vi "BatteryCal FTS.vi"() -> ()   [LabVIEW 2013]
uses:
  Controls/Gen2 FT states.ctl
  SubVI/ESTOP CONTROL.ctl
  Controls/InfoPacket.ctl
  Controls/Target RF Channel.ctl
  <vilib>/Utility/error.llb/DialogType.ctl
  Controls/LocalVars.ctl
  Controls/Iniial Device Programming.ctl
  SubVI/ProgramStageControl.ctl
  Controls/Batt Cap Steps.ctl
  Controls/Support Script.ctl
  Controls/Serial Table.ctl
  Controls/Device Information.ctl
  Controls/Loading.ctl
  Controls/Load Step.ctl
  Controls/Mark10 Config.ctl
  Controls/PID parameters.ctl
  Controls/Channels.ctl
  RxTx/XceiverStates.ctl
  RxTx/XceiverCmds.ctl
  Controls/Mark10 states.ctl
  Controls/Gen2 FT Globals.vi
  <vilib>/Utility/file.llb/Write To Spreadsheet File (I64).vi
  <vilib>/Utility/config.llb/Write Key (String).vi
  <vilib>/Utility/config.llb/NI_LVConfig.lvlib
panel:
  out "Transceiver Channel:":u8
  out "DUT Serial Number":u32
  in  "A2 Delay (ms)":i16=500 min=-1 step=1
  in  "Save EEPROM Data":bool caption="DevOFF"
  out "EEPROM Data":i32[][](array[numeric])
  in  "Close Xsceiver":bool
  in  "Scan Channels":bool caption="DevOFF"
  in  "Clear Message":bool
  out "Rev String":string
  in  "Target Channel:":T1="5"
  in  "mSec":u8=1 min=1 max=50 step=1
  in  "Set Wndow":bool caption="DevOFF"
  in  "Get Window":bool caption="DevOFF"
  out "ADBatt":u16
  out "BattVolts":dbl format="%_3g"
  out "BatteryCapState":i8
  out "Batt280":i32
  out "Batt310":i32
  out "Accelerometer sample size":i32
  out "Base Accels":dbl[][](array[numeric])
  out "Six Plane Accels":dbl[][](array[numeric])
  in  "Reset Device":bool=TRUE
  in  "CaptureButton":bool
  out "Message":string
  out "AssemScore":i32
  out "PCB Score":i32
  out "GAINC Reprogram?":bool
  out "Three Failed Tests":dbl
  in  "Mark-10 COM Port":refnum<visa-resource-name>="COM1"
  in  "Eng-Result# :":u32 max=268435455
  in  "Start Channel:":string(combo)="3"
  in  "Brand:":string(combo)
  in  "DeviceType:":string(combo)="SYK-TRCR01"
  out "Device Parameters":T2 {"ASICtrim" format="%02x"}
  out "Device ON?":bool
  in  "Start":bool
  out "SoftwareVersion":string="SW-03004-002"
  out "Adj.Data":dbl[](array[numeric])
  out "RawData":u16[](array[numeric]) caption="RawData\n      S3         S4           S5         S6         S7          S8          S9          B"
  in  "Operator":string caption="Operator Name:"
  out "DeviceID:":u32
  out "Current Time:":timestamp=timestamp(3438190648.7035365 s since 1904-01-01) format="%<%I:%M:%S %p\n%m/%d/%Y>T"
  in  "Lot#:":u32
  in  "ClearBuffer":bool
  in  "Exit":bool
  in  "Estop":T3
  in  "Shutdown Dev":bool caption="DevOFF"
  out "Test Result":bool
  in  "States":T4=enum."Initialization"
  out "error out":errorcluster
  # "lbs"
  # "inch"
  # "Mark-10"
  # "Engineering Panel"
  # "OrthoSensor Battery Calibration"
  # "System Messages"
  # "Target Loads\n(lbs)"
  # "Gauge Loads\n(lbs)"
  # "Total Device \nLoads (lbs)"
  # "Device Loads"
  # "Errors"
  # "A (lbs)                  B (lbs)"
  # "A (lbs)                 B (lbs)"
  # "Device"
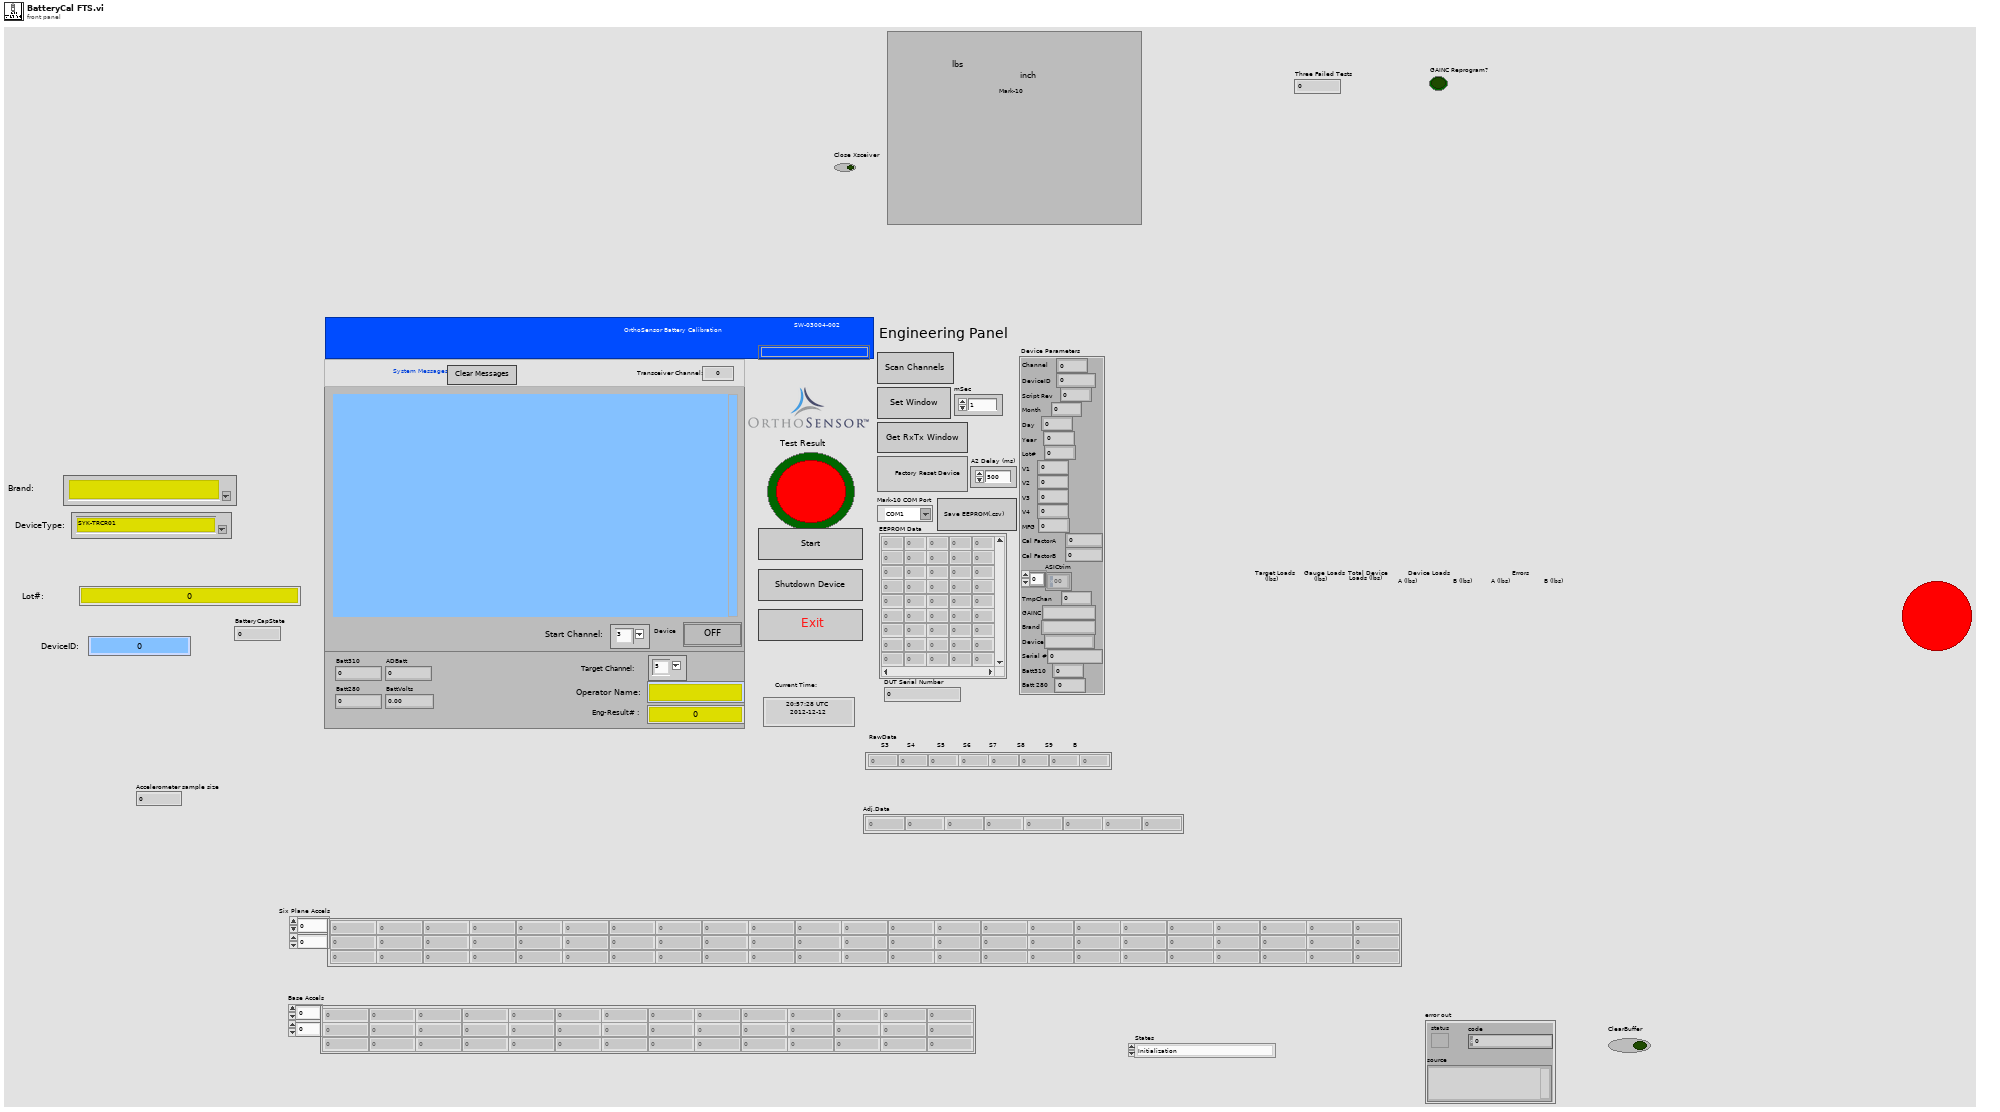
[diagram p1: front panel]
types:
  T1 = typedef "Target RF Channel.ctl" = string
  T2 = typedef "InfoPacket.ctl" = cluster{"Channel":u8, "DeviceID":u32, "Script Rev":u8, "Month":u8, "Day":u8, "Year":u8, "Lot#":u32, "V1":u16, "V2":u16, "V3":u16, "V4":u16, "MFG":u8, "Cal FactorA":u8, "Cal FactorB":u8, "ASICtrim":u8[], "TmpChan":u8, "GAINC":string, "Brand":string, "Device":string, "Serial #":u64, "Batt310":u16, "Batt 280":u16}
  T3 = typedef "ESTOP CONTROL.ctl" = bool
  T4 = typedef "Gen2 FT states.ctl" = enum16{"---------SETUP-------", "Initialization", "Read Support Data", "Initialize Mark-10", "Initialize Transceiver", "------UTILITIES------", "Change DUT Channel", "Find RxTx Window", "Reset Device", "Scan Channels", "Read Serial Lookup", "Shutdown Device", "ESTOP", "--------USER---------", "Timeout", "-----PROGRAM-----", "Program Device", "------MARK10--------", "Go Home", "MoveUp", "MoveDown", "Goto Load", "Goto Position", "Stop Motor", "---------TESTS--------", "Start Test", "Angle Test", "Load Test", "Load Accuracy Test", "Battery Test", "------RESULTS-------", "End Test", "Display Result", "--------EXIT--------", "Exit"}
  T5 = typedef "XceiverStates.ctl" = enum16{"Initialize", "Rx", "Tx", "Raw Mode", "Clear Buffer", "ClearEcho", "Read Buffer", "Close"}
  T6 = typedef "LocalVars.ctl" = cluster{"Message":string, "Homed?":bool, "NextState":T4, "G.Load":dbl, "G.Position":dbl, "Load#":i32, "[G.Loads]":dbl[], "[TotalLoads]":dbl[], "[Errors]":dbl[][], "ZeroWait":u32, "Results":dbl[], "DwellWait":bool, "Test Result":bool, "[CondyleLoads]":dbl[][], "[Max]":dbl[], "[Min]":dbl[], "Valid String?":bool, "ScanTime":timestamp, "ScannedString":string, "LabelDevID":u32, "MfgDate":timestamp, "[EEPROM Cmds]":u8[][], "[CalData]":u8[][], "[A/Ds]":dbl[][], "[A/Dmax]":dbl[], "[A/Dmin]":dbl[], "BattMax":dbl, "BattMin":dbl, "DwellTime":i32, "PendingDeviceType":string, "Zero G.load":dbl, "GAINC Value":string, "Programming Step":T7, "Front Panel Program?":bool, "Final Program?":bool, "PCB Score":i32, "AssyScore":i32, "Pass/Fail #":string, "Result String":string, "Programming Mode":T8, "Angle Test Step":enum16{"Initialize", "Get X", "Get Y", "Get Z", "Next Test"}, "Accel Values":dbl[][], "Shutdown Counter":u32, "V1":i32, "V2":i32, "V3":i32, "V4":i32, "EEPROM Data":i32[][], "Counter":i32, "Page#":i32, "Timer":timestamp, "Use Mark10?":bool, "Eng-Result#":u32, "DUT Serial #":i32, "Scroll Message?":bool, "Clear Message":bool, "Batt Test Step ":T9, "RXTX Window Found?":bool, "Shutdown First Call?":bool, "A2 Delay (msec)":i16, "Support Script":T10, "Serial Table":T11, "Target Information":T12, "Operator":string, "COM Port":string, "Config Path":path, "Tx Array":u8[], "DUT Parameters":T2, "FTS Main?":bool, "Loading":T13, "Software Version":string, "Correction Factor":string, "Second Load Test":bool, "Acc Loads":dbl[][], "Mark10 Config":T15, "Channels":T17, "Channel EEPROM":i32[][], "Load Notes":string[], "Engr Log?":bool, "Time":timestamp[], "Program Retry":bool, "Operator Channel":string, "Target Channel ":string, "New Data Program":bool}
  T7 = typedef "Iniial Device Programming.ctl" = enum16{"Load EEPROM", "Send First A1", "Send EEPROM", "Send A1", "Check EEPROM Echo", "Verify transmission", "Programming Successful", "Programming Failed"}
  T8 = typedef "ProgramStageControl.ctl" = enum16{"Initial Program", "GainC", "Scales"}
  T9 = typedef "Batt Cap Steps.ctl" = enum16{"Initialize", "Collect 2.8 Volts", "Collect 3.1 Volts", "Check Results"}
  T10 = typedef "Support Script.ctl" = cluster{"Script #":string, "Script Revision":string, "[OEMs]":string[], "[[DeviceTypes]]":string[][], "[[DeviceTypesVals]]":u16[][], "[[List of Errors]]":string[][], "Default GAINC":string, "[[ASICtrims]]":u8[][], "ID For Echo":string, "Condyle A CalFactor":i32, "Condyle B CalFactor":i32, "[OEMs Prefix]":string[], "Packet ID 18":string, "[[Force Table Load Test]]":dbl[][], "[[Force Table AccurTest]]":dbl[][]}
  T11 = typedef "Serial Table.ctl" = cluster{"Serial File Path":path, "[[Serial Lookup Table]]":string[][], "Serial Device Info":string[], "Valid Serial?":bool}
  T12 = typedef "Device Information.ctl" = cluster{"Target Brand":string, "Target DeviceType":string, "Target Serial#":i32, "Target Lot#":u32, "Target DevID":u32, "Target Channel":u8}
  T13 = typedef "Loading.ctl" = cluster{"[Forces]":dbl[], "[Dwell]":dbl[], "Loading Step":T14}
  T14 = typedef "Load Step.ctl" = enum16{"Initialize Test", "Go Home", "Detect Dev Surface", "Wait to zero Device", "Zero Device", "Do Test", "Test Result"}
  T15 = typedef "Mark10 Config.ctl" = cluster{"H2S%":dbl[], "H2S Speed":dbl[], "H to S":dbl, "Home Speed":dbl, "LoadWin":dbl, "Load Speed":dbl, "PID":T16}
  T16 = typedef "PID parameters.ctl" = cluster{"Kp":dbl, "Kd":dbl, "Ki":dbl}
  T17 = typedef "Channels.ctl" = cluster{"Transceiver Ch":u8, "Operating Ch":u8, "Start Ch":u8}
  T18 = typedef "DialogType.ctl" = u16
  T19 = enum8{"Enabled", "Disabled", "Disabled and Grayed Out"}
  T20 = enum16{"None", "On Hover", "On Key Focus", "On Hover or Key Focus"}
  T21 = typedef "Mark10 states.ctl" = enum16{"Initialize", "Go Home", "Move Up", "Move Down", "Stop @ Load", "Read Status", "Goto Position", "Goto Device Surface", "Stop Motor", "Shutdown", "Exit"}
  T22 = typedef "XceiverCmds.ctl" = enum8{"Get Window", "Set Window", "Load&Xmit", "Find Window", "Load CC1101", "Blink LED1", "Blink LED2", "Gen2 Mode", "Request Rev", "Gen2 Mode & Req Rev", "Load Device Settings", "Reset Xceiver", "Set Channel", "Read Channel"}
  T23 = cluster{"Shift":bool, "Ctrl":bool, "Alt":bool, "Cmd":bool, "Opt":bool}
  T24 = typedef "Scanned Data.ctl" = cluster{"DeviceID":u32, "Mfg Date":timestamp, "ScannedIn":bool, "Lot#":u32}
  T25 = typedef "LVRectTypeDef.ctl" = cluster{"Left":i16, "Top":i16, "Right":i16, "Bottom":i16}
  T26 = typedef "DeviceInfo.ctl" = cluster{"DevInfo":T2, "Mfg Date":timestamp, "[CalData]":u8[][], "[DevData]":u8[], "GotCal":bool, "CustomCal?":bool, "Packet#":i32}
  T27 = typedef "NI_LVConfig.lvlib/Config Data RefNum.ctl" = refnum<k1>
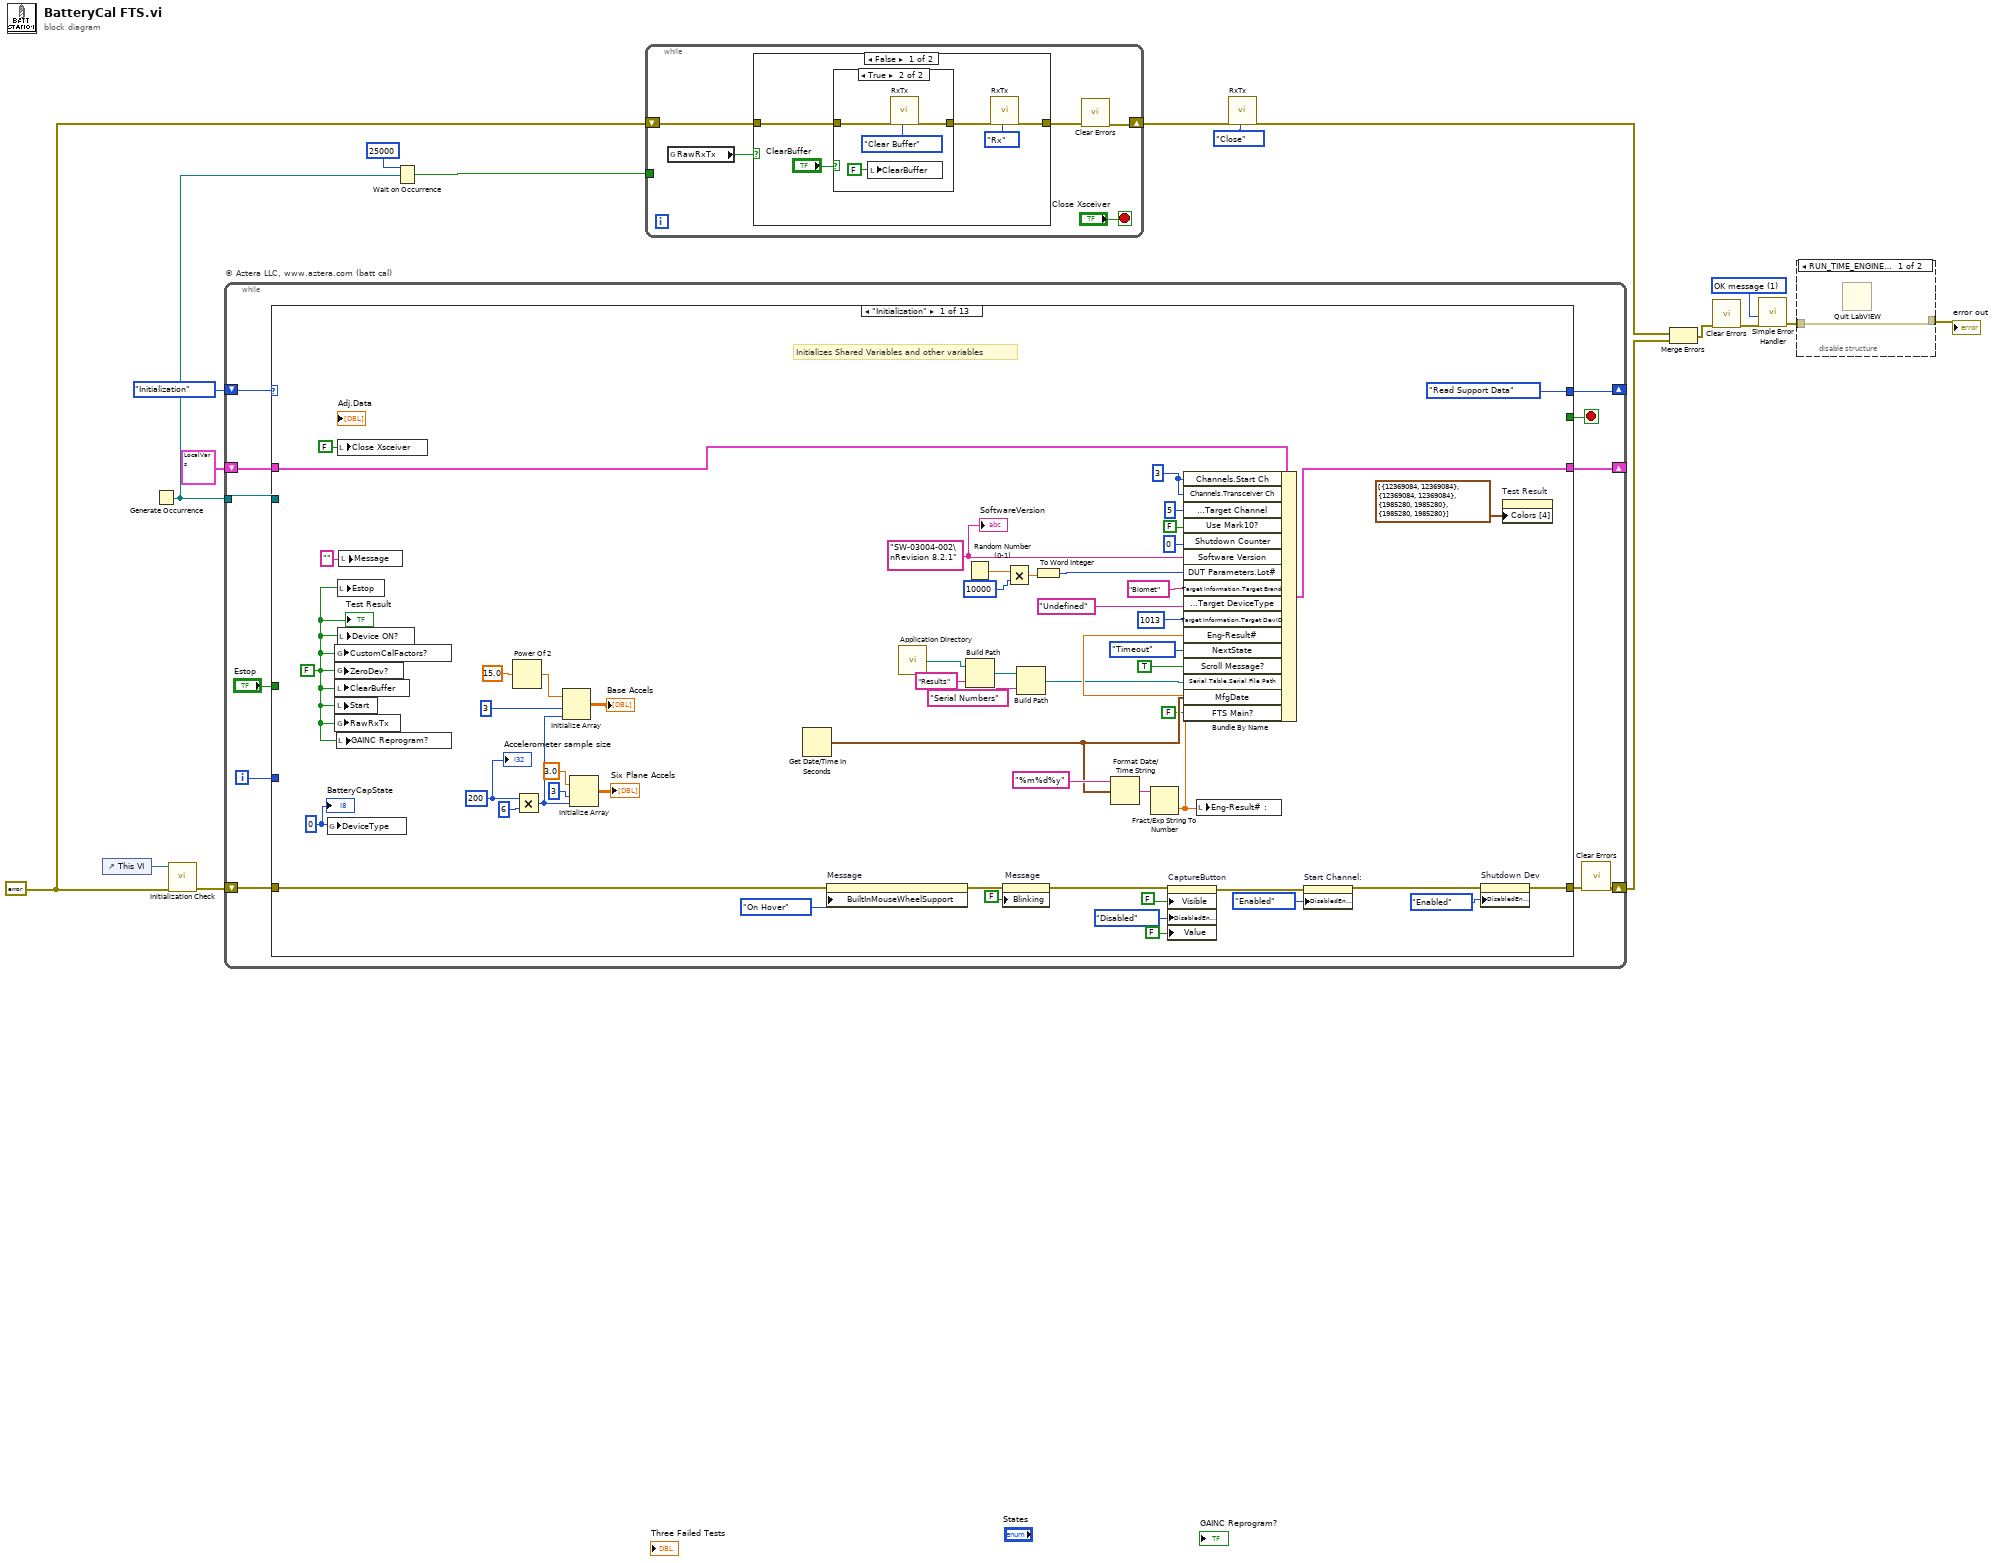
[diagram p0: block diagram]
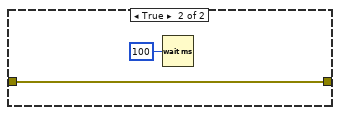
[diagram p3: hidden frame]
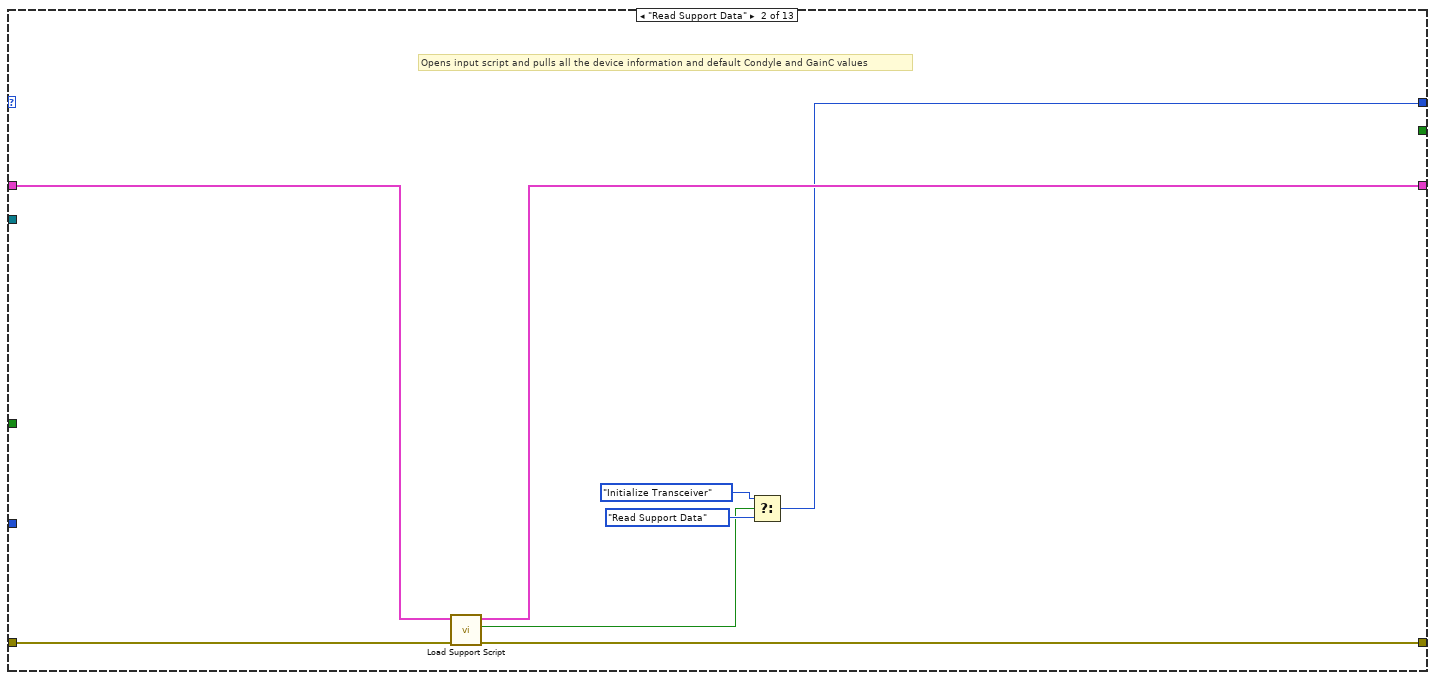
[diagram p5: hidden frame]
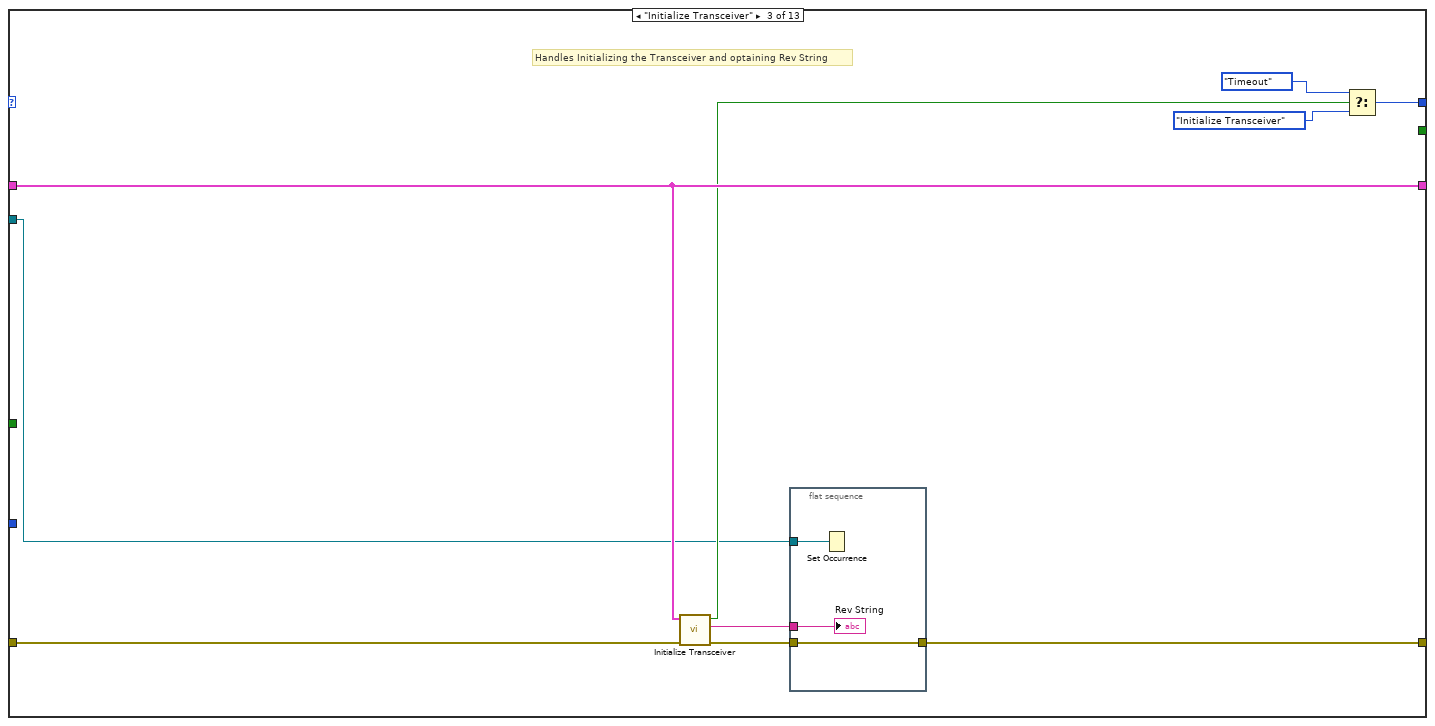
[diagram p6: hidden frame]
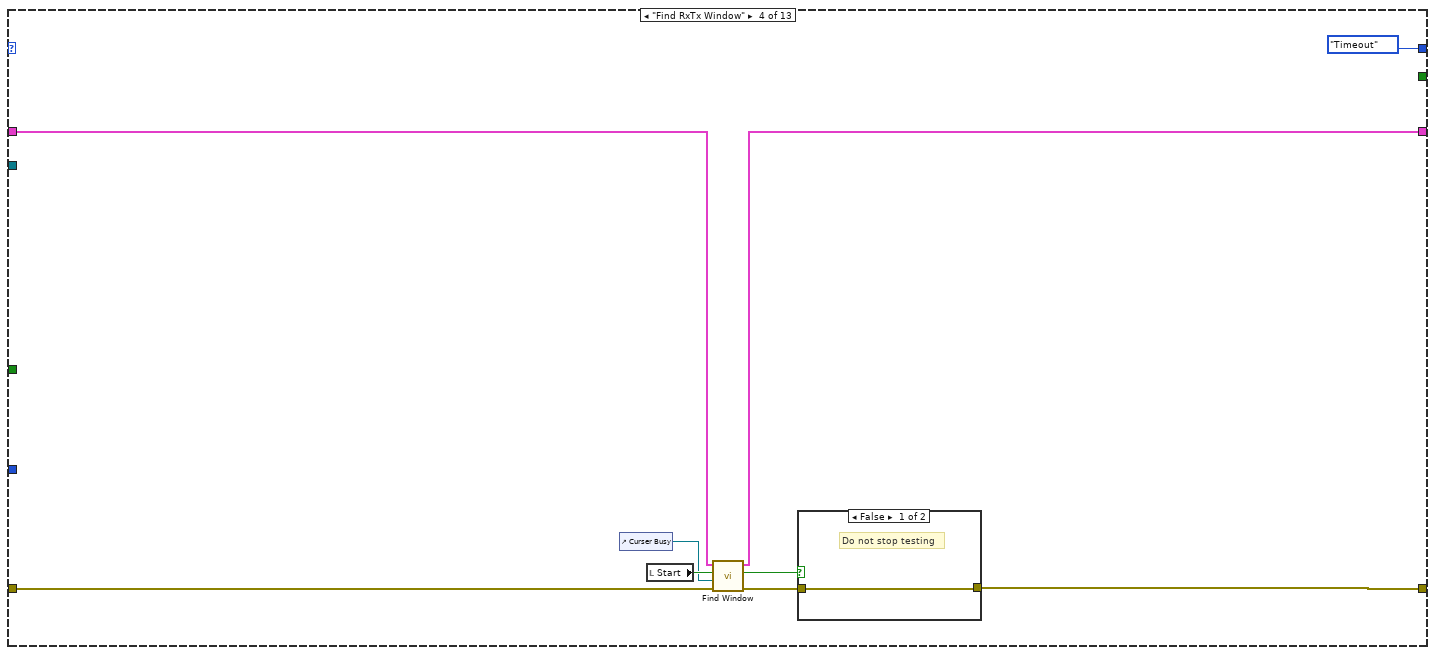
[diagram p7: hidden frame]
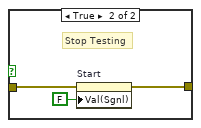
[diagram p8: hidden frame]
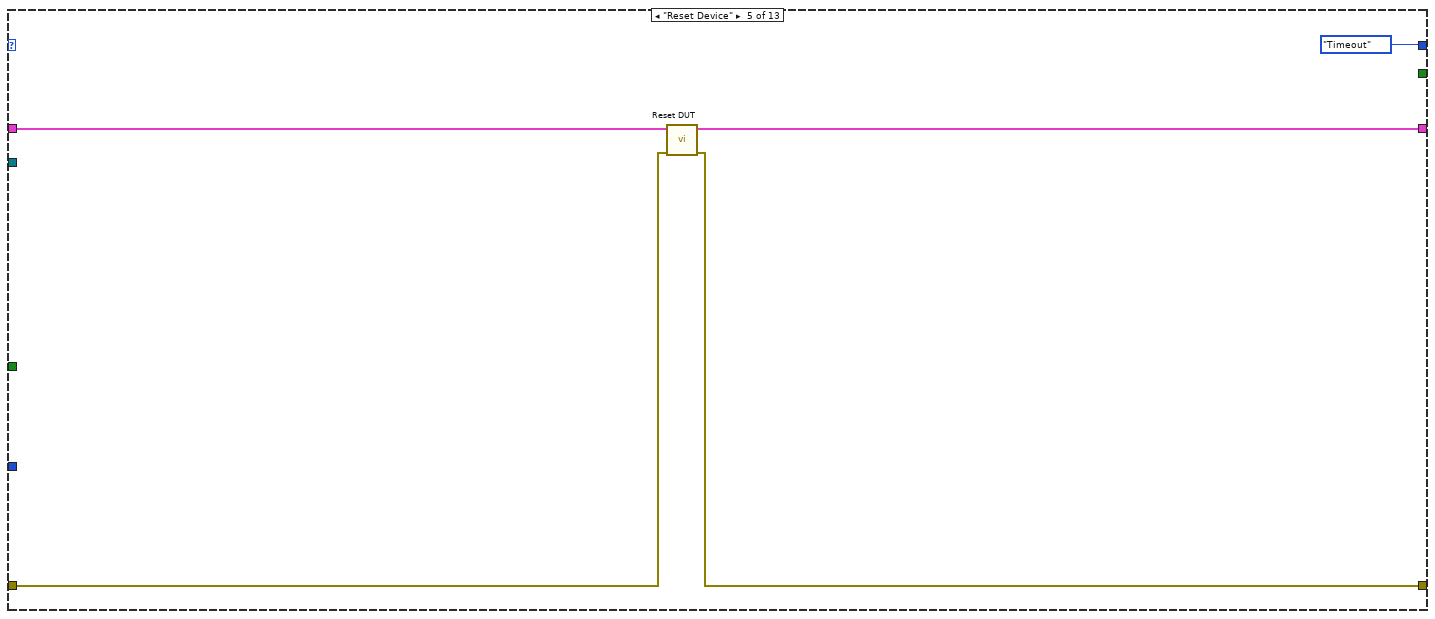
[diagram p9: hidden frame]
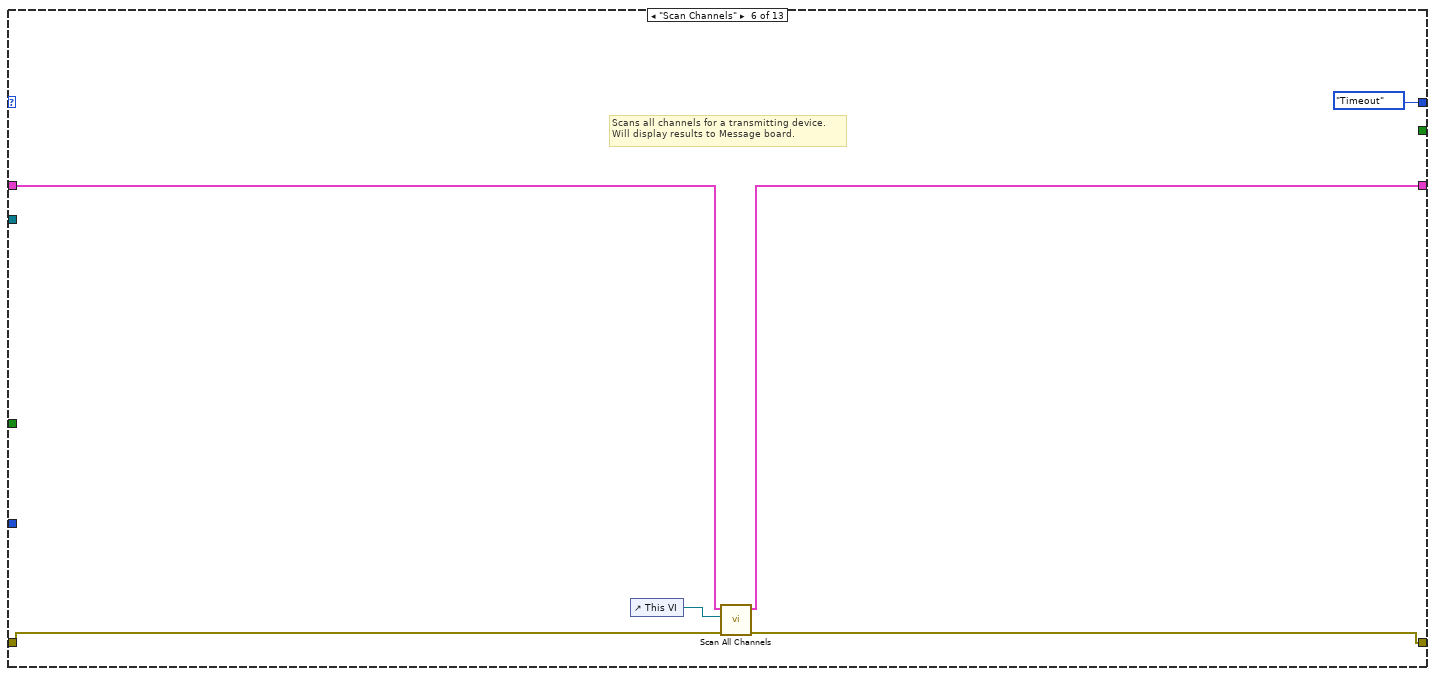
[diagram p10: hidden frame]
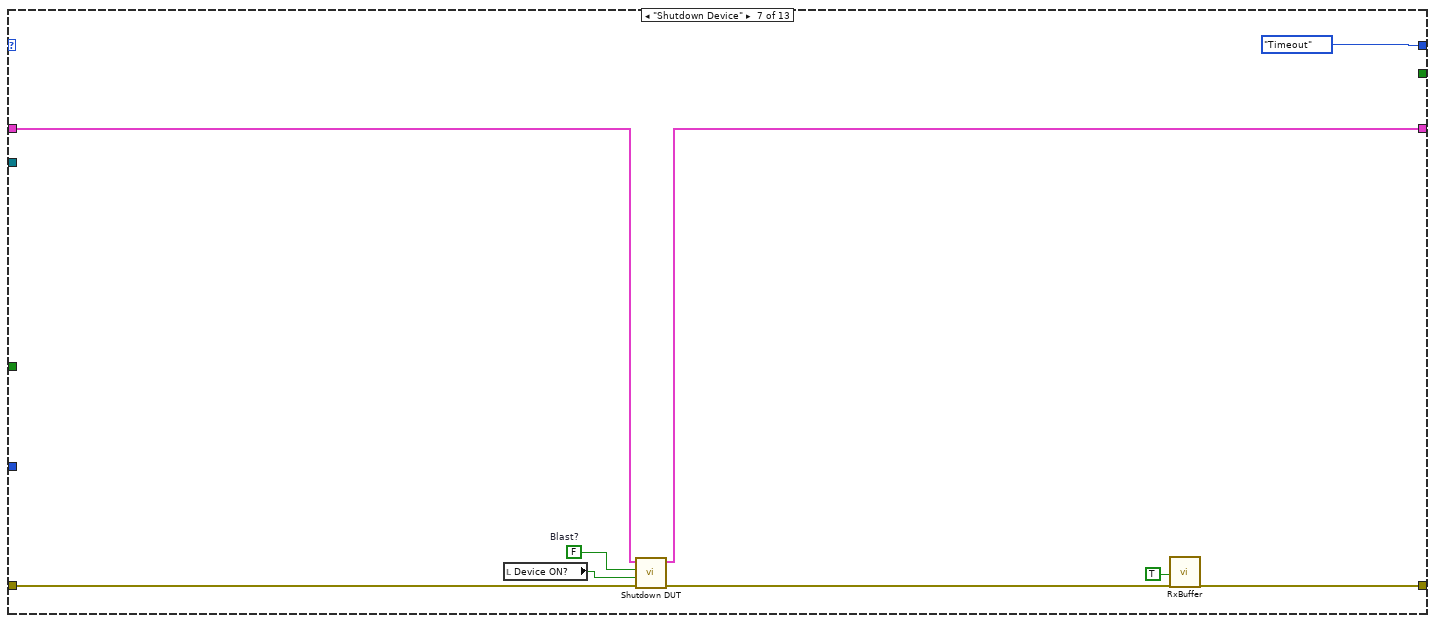
[diagram p11: hidden frame]
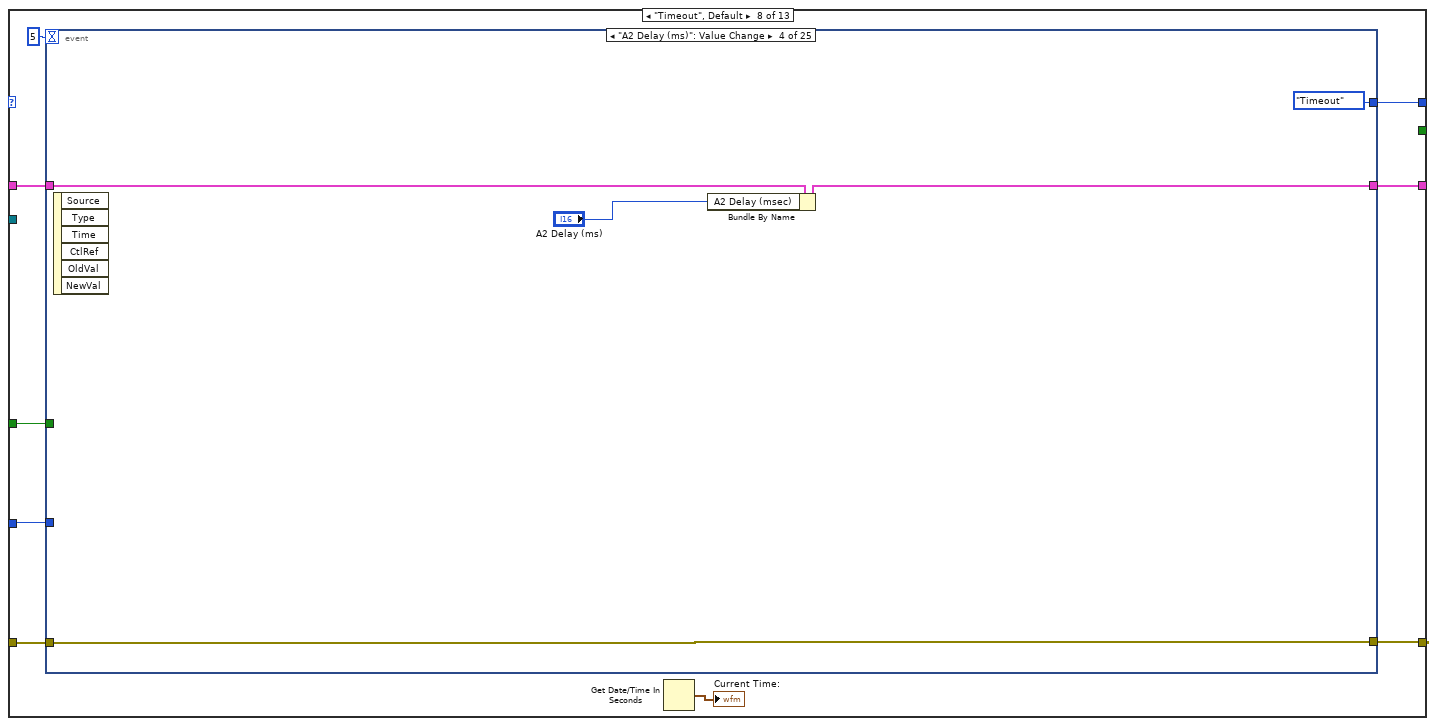
[diagram p12: hidden frame]
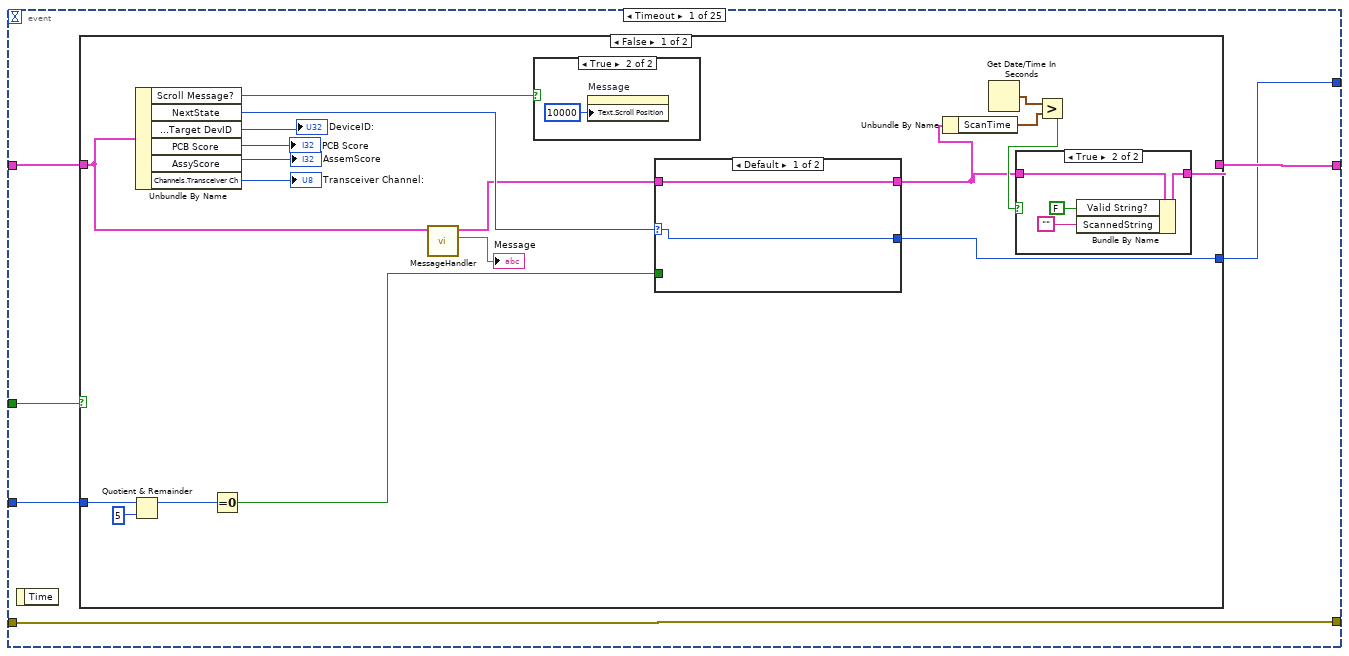
[diagram p13: hidden frame]
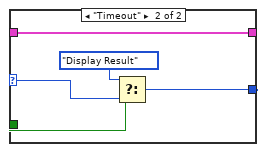
[diagram p16: hidden frame]
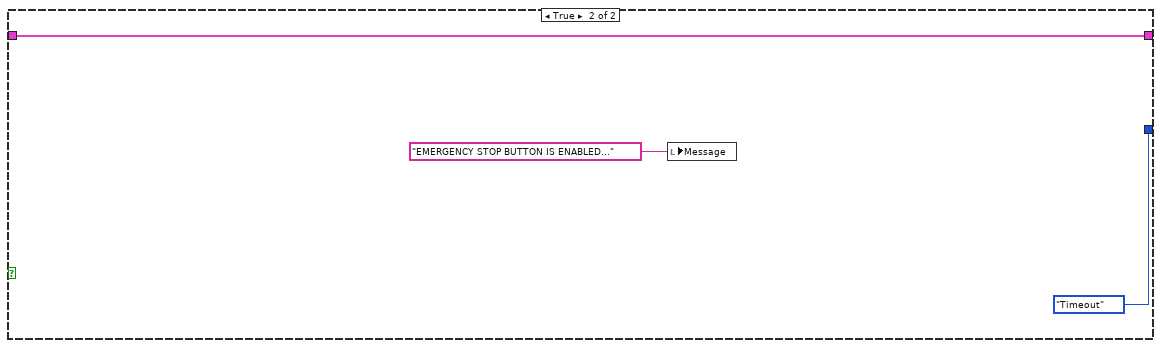
[diagram p17: hidden frame]
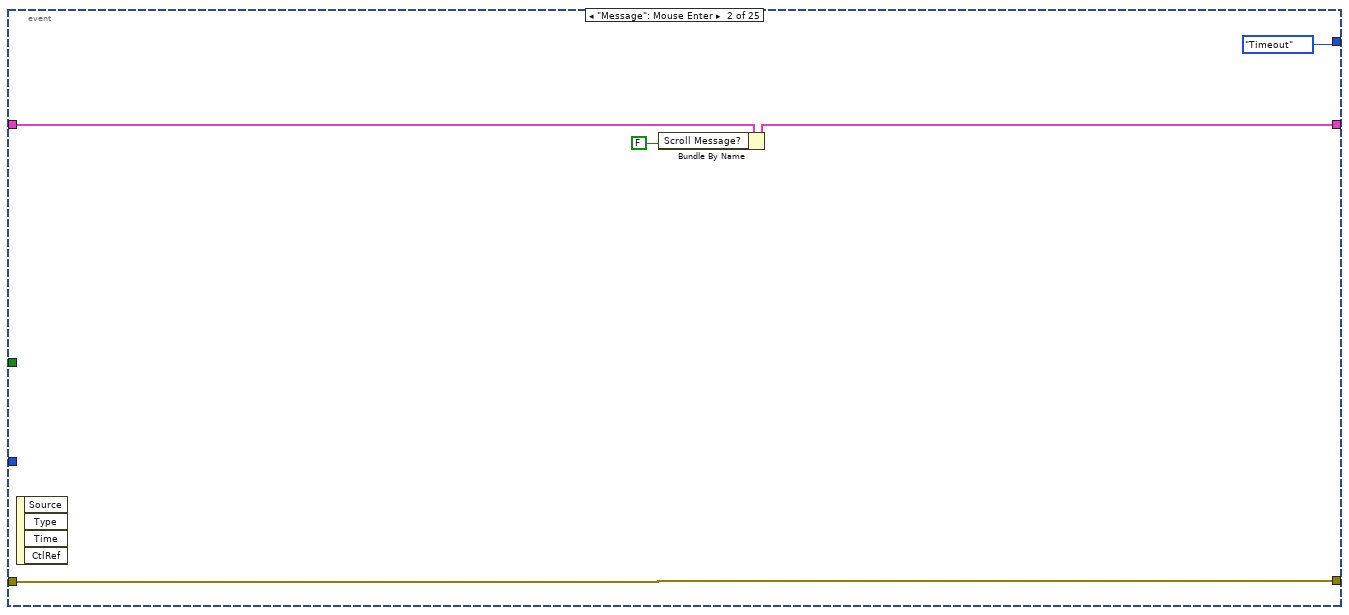
[diagram p18: hidden frame]
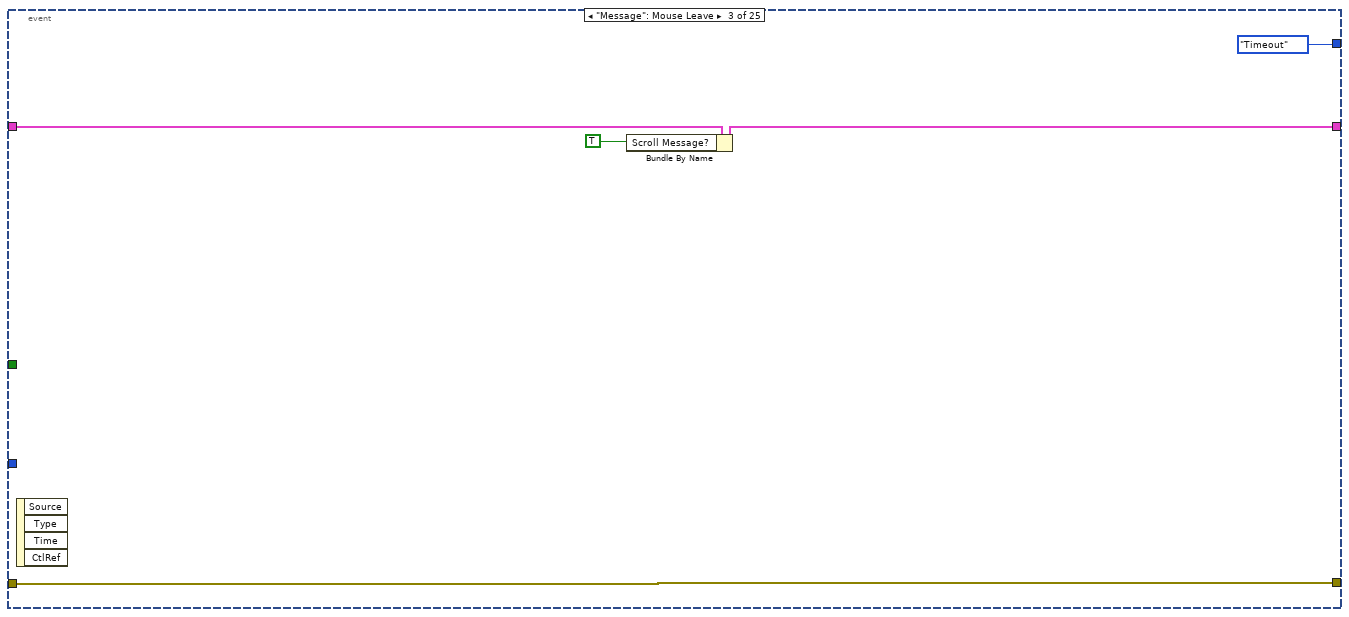
[diagram p19: hidden frame]
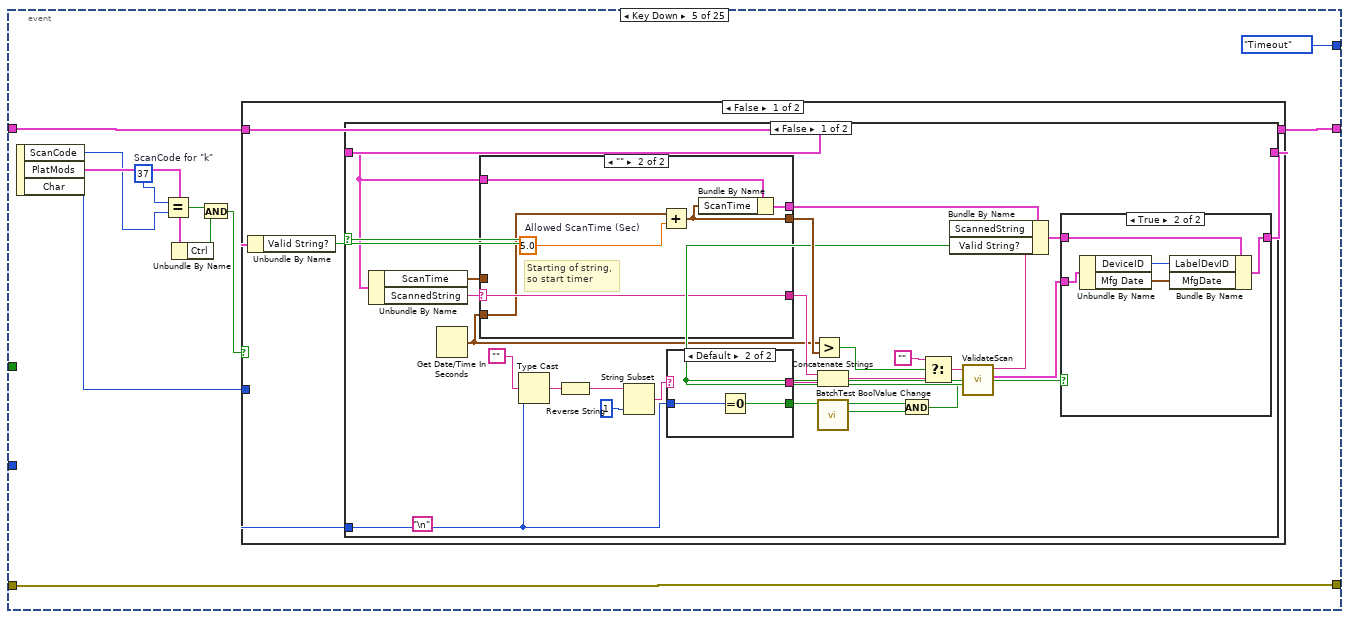
[diagram p20: hidden frame]
diagram:
  w12 = T18 1 items=["no dialog", "OK message", "continue or stop message", "OK message + warnings", "continue/stop + warnings"] ("type of dialog (OK msg:1)")
  w3 = errorcluster {"status"=FALSE, "code"=0, "source"=""} ("error in (no error)")
  n1 = control-ref of="This VI"() -> (w7:refnum<vi>)
  n2 = Generate Occurrence() -> (w15:refnum<k4>)
  n3 = call "Initialization Check.vi"("error in (no error)"=w3, "VI in"=w7) -> ("error out"=w6:errorcluster)  [unwired: 9 in]
  n4 = while "© Aztera LLC, www.aztera.com (batt cal)" {
    shift-right: [w21] -> _
    shift-left: T6 {"Message"="", "Homed?"=FALSE, "NextState"=enum."Scan Channels", "G.Load"=0.0, "G.Position"=0.0, "Load#"=0, "[G.Loads]"=[], "[TotalLoads]"=[], "[Errors]"=[], "ZeroWait"=0, "Results"=[], "DwellWait"=FALSE, "Test Result"=FALSE, "[CondyleLoads]"=[], "[Max]"=[], "[Min]"=[], "Valid String?"=FALSE, "ScanTime"=timestamp(0 s since 1904-01-01), "ScannedString"="", "LabelDevID"=0, "MfgDate"=timestamp(0 s since 1904-01-01), "[EEPROM Cmds]"=[], "[CalData]"=[], "[A/Ds]"=[], "[A/Dmax]"=[], "[A/Dmin]"=[], "BattMax"=0.0, "BattMin"=0.0, "DwellTime"=0, "PendingDeviceType"="", "Zero G.load"=0.0, "GAINC Value"="", "Programming Step"=enum."Load EEPROM", "Front Panel Program?"=FALSE, "Final Program?"=FALSE, "PCB Score"=0, "AssyScore"=0, "Pass/Fail #"="", "Result String"="", "Programming Mode"=enum."Initial Program", "Angle Test Step"=enum."Initialize", "Accel Values"=[], "Shutdown Counter"=0, "V1"=0, "V2"=0, "V3"=0, "V4"=0, "EEPROM Data"=[], "Counter"=0, "Page#"=0, "Timer"=timestamp(0 s since 1904-01-01), "Use Mark10?"=FALSE, "Eng-Result#"=0, "DUT Serial #"=0, "Scroll Message?"=FALSE, "Clear Message"=FALSE, "Batt Test Step "=enum."Initialize", "RXTX Window Found?"=FALSE, "Shutdown First Call?"=FALSE, "A2 Delay (msec)"=0, "Support Script"={"Script #"="", "Script Revision"="", "[OEMs]"=[], "[[DeviceTypes]]"=[], "[[DeviceTypesVals]]"=[], "[[List of Errors]]"=[], "Default GAINC"="", "[[ASICtrims]]"=[], "ID For Echo"="", "Condyle A CalFactor"=0, "Condyle B CalFactor"=0, "[OEMs Prefix]"=[], "Packet ID 18"="", "[[Force Table Load Test]]"=[], "[[Force Table AccurTest]]"=[]}, "Serial Table"={"Serial File Path"=path "", "[[Serial Lookup Table]]"=[], "Serial Device Info"=[], "Valid Serial?"=FALSE}, "Target Information"={"Target Brand"="", "Target DeviceType"="", "Target Serial#"=0, "Target Lot#"=0, "Target DevID"=0, "Target Channel"=0}, "Operator"="", "COM Port"="", "Config Path"=path "", "Tx Array"=[], "DUT Parameters"={"Channel"=0, "DeviceID"=0, "Script Rev"=0, "Month"=0, "Day"=0, "Year"=0, "Lot#"=0, "V1"=0, "V2"=0, "V3"=0, "V4"=0, "MFG"=0, "Cal FactorA"=0, "Cal FactorB"=0, "ASICtrim"=[], "TmpChan"=0, "GAINC"="", "Brand"="", "Device"="", "Serial #"=0, "Batt310"=0, "Batt 280"=0}, "FTS Main?"=FALSE, "Loading"={"[Forces]"=[], "[Dwell]"=[], "Loading Step"=enum."Initialize Test"}, "Software Version"="", "Correction Factor"="", "Second Load Test"=FALSE, "Acc Loads"=[], "Mark10 Config"={"H2S%"=[], "H2S Speed"=[], "H to S"=0.0, "Home Speed"=0.0, "LoadWin"=0.0, "Load Speed"=0.0, "PID"={"Kp"=0.0, "Kd"=0.0, "Ki"=0.0}}, "Channels"={"Transceiver Ch"=0, "Operating Ch"=0, "Start Ch"=0}, "Channel EEPROM"=[], "Load Notes"=[], "Engr Log?"=FALSE, "Time"=[], "Program Retry"=FALSE, "Operator Channel"="", "Target Channel "="", "New Data Program"=FALSE} ("State-machine Local Variables") -> [w26]
    shift-right: [w22] -> w17
    shift-left: w6 -> [w27]
    tunnel: w15 -> [w24]
    shift-right: [w19] -> _
    shift-left: Gen2_FT_states."Initialization" ("Current State Out") -> [w18]
    i -> [w25]
    stop <- w20 stop-if-true
    n5 = case shown="\"Initialization\"" w18 {
      tunnel: [w43 w86 w92 w108 w119 w127 w130 w139 w608 w611 w708 w732 w759] -> w28
      tunnel: w27 -> [w33 w91 w101 w107 w120 w128 w135 w140 w609 w612 w707 w744 w765]
      tunnel: w26 -> [w78 w90 w96 w113 w122 w124 w136 w143 w606 w614 w710 w723 w764]
      tunnel: [Gen2_FT_states."Read Support Data" ("Current State Out") w87 w98 Gen2_FT_states."Timeout" ("Current State Out") Gen2_FT_states."Timeout" ("Current State Out") Gen2_FT_states."Timeout" ("Current State Out") Gen2_FT_states."Timeout" ("Current State Out") w144 Gen2_FT_states."Timeout" ("Current State Out") Gen2_FT_states."Timeout" ("Current State Out") Gen2_FT_states."Timeout" ("Current State Out") Gen2_FT_states."Timeout" ("Current State Out") Gen2_FT_states."Exit" ("Current State Out")] -> w19
      tunnel: w25 -> [_ _ _ _ _ _ _ w142 _ _ _ _ _]
      tunnel: w24 -> [_ _ w94 _ _ _ _ _ _ _ _ _ _]
      tunnel: "Estop" -> [_ _ _ _ _ _ _ w141 _ _ _ _ _]
      tunnel: [w46 w89 w96 w105 w118 w126 w132 w138 w605 w615 w702 w723 w763] -> w21
      tunnel: [_ _ _ _ _ _ _ _ _ _ _ _ TRUE] -> w20
      frame "Initialization" {
        w29 = u8 3 ("Current Channel")
        w55 = "SW-03004-002\nRevision 8.2.1" ("SoftwareVersion")
        w67 = 200
        w76 = u32 0 ("Lot Number")
        w45 = FALSE ("Exit")
        # "Initializes Shared Variables and other variables"
        n6 = global write "Gen2 FT Globals.vi" "DeviceType"(w76) -> ()
        n7 = global write "Gen2 FT Globals.vi" "CustomCalFactors?"(w45) -> ()
        n8 = global write "Gen2 FT Globals.vi" "ZeroDev?"(w45) -> ()
        n9 = local write "ClearBuffer"(w45) -> ()
        n10 = local write "Start"(w45) -> ()
        n11 = global write "Gen2 FT Globals.vi" "RawRxTx"(w45) -> ()
        n12 = local write "GAINC Reprogram?"(w45) -> ()
        n13 = local write "Close Xsceiver"(FALSE ("Close Xsceiver")) -> ()
        n14 = local write "Estop"(w45) -> ()
        n15 = local write "Device ON?"(w45) -> ()
        n16 = local write "Message"("" ("Message")) -> ()
        n17 = Power Of 2(x=15.0) -> (2^x=w75:dbl)
        n18 = Multiply(x=w67, y=6) -> (x*y=w66:i32)
        n19 = Initialize Array(w75, 3, w66) -> (→"Base Accels":dbl[][])
        n20 = Initialize Array(3.0, 3, w66) -> (→"Six Plane Accels":dbl[][])
        n21 = Get Date/Time In Seconds() -> (seconds since 1Jan1904=w32:timestamp)
        n22 = property on="Message" class="Str"(error in=w33, "BuiltInMouseWheelSupport"=T20."On Hover" ("Built-In Mouse Wheel Support")) -> (error out=w77:errorcluster)  [unwired: 1 in, 1 out]
        n23 = call <vilib>:"Application Directory.vi"() -> ("Application Directory"=w38:path)
        n24 = Random Number (0-1)() -> (number: 0 to 1=w54:dbl)
        n25 = Build Path(base path=w38, name or relative path="Results") -> (appended path=w36:path)
        n26 = property on="Message" class="Str"(error in=w77, "Blinking"=FALSE) -> (error out=w56:errorcluster)  [unwired: 1 in, 1 out]
        n27 = Multiply(x=w54, y=10000) -> (x*y=w53:dbl)
        n28 = Build Path(base path=w36, name or relative path="Serial Numbers") -> (appended path=w34:path)
        n29 = To Word Integer(number=w53) -> (16bit integer=w52:i16)
        n30 = Format Date/Time String(time format string (%c)="%m%d%y", seconds (now)=w32) -> (date/time string=w57:string)  [unwired: 1 in]
        n31 = Fract/Exp String To Number(string=w57) -> (number=w50:dbl)  [unwired: 3 in, 1 out]
        n32 = property on="CaptureButton" class="Bool (strict)"(error in=w56, "Visible"=FALSE, "DisabledEnum"=T19."Disabled" ("Disabled"), "Value"=FALSE ("CaptureButton")) -> (error out=w60:errorcluster)  [unwired: 1 in, 1 out]
        n33 = Bundle By Name(cluster=w78, "Channels.Start Ch"=w29, "Channels.Transceiver Ch"=w29, "Target Information.Target Channel"=u8 5 ("Target Channel"), "Use Mark10?"=FALSE ("FTS Main?"), "Shutdown Counter"=u32 0, "Software Version"=w55, "DUT Parameters.Lot#"=w52, "Target Information.Target Brand"="Biomet", "Target Information.Target DeviceType"="Undefined", "Target Information.Target DevID"=1013, "Eng-Result#"=w50, "NextState"=Gen2_FT_states."Timeout", "Scroll Message?"=TRUE, "Serial Table.Serial File Path"=w34, "MfgDate"=w32, "FTS Main?"=FALSE) -> (w46:T6)
        n34 = local write "Eng-Result# :"(w50) -> ()
        n35 = property on="Start Channel:" class="CmbBox"(error in=w60, "DisabledEnum"=T19."Enabled" ("Disabled")) -> (error out=w44:errorcluster)  [unwired: 1 in, 1 out]
        n36 = property on="Shutdown Dev" class="Bool"(error in=w44, "DisabledEnum"=T19."Enabled" ("Disabled")) -> (error out=w43:errorcluster)  [unwired: 1 in, 1 out]
        n37 = property on="Test Result" class="Bool (strict)"("Colors [4]"=cluster{u32, u32}[] [{12369084, 12369084}, {12369084, 12369084}, {1985280, 1985280}, {1985280, 1985280}]) -> ()  [unwired: 2 in, 2 out]
        "BatteryCapState" <- w76
        "Accelerometer sample size" <- w67
        "SoftwareVersion" <- w55
        "Test Result" <- w45
      }
      frame "Read Support Data" {
        # "Opens input script and pulls all the device information and default Condyle and GainC values"
        n38 = call "Load Support Script.vi"("error in (no error)"=w91, "Data In"=w90) -> ("error out"=w86:errorcluster, "Done?"=w84:bool, "Data Out"=w89:T6)  [unwired: 7 in]
        n39 = Select(t=Gen2_FT_states."Initialize Transceiver" ("Current State Out"), s=w84, f=Gen2_FT_states."Read Support Data") -> (s? t:f=w87:T4)
      }
      frame "Initialize Transceiver" {
        # "Handles Initializing the Transceiver and optaining Rev String"
        n40 = call "Initialize Transceiver.vi"("error in (no error)"=w101, "State-machine Local Variables"=w96) -> ("error out"=w93:errorcluster, "Rev String"=w100:string, "Initialized?"=w95:bool)  [unwired: 7 in]
        n41 = flat-sequence {
          tunnel: w100 -> [w104]
          tunnel: w94 -> [w103]
          tunnel: w93 -> [w102]
          tunnel: [w102] -> w92
          frame #0 {
            n42 = Set Occurrence(w103) -> ()
            "Rev String" <- w104
          }
        }
        n43 = Select(t=Gen2_FT_states."Timeout" ("Current State Out"), s=w95, f=Gen2_FT_states."Initialize Transceiver") -> (s? t:f=w98:T4)
      }
      frame "Find RxTx Window" {
        n44 = control-ref of="Curser Busy"() -> (w106:refnum<vi>)
        n45 = local read "Start"() -> (w111:bool)
        n46 = call "Find Window.vi"("error in (no error)"=w107, "This VI"=w106, "Testing?"=w111, "Main Data"=w113) -> ("error out"=w109:errorcluster, "Stop Testing?"=w110:bool, "Main Data"=w105:T6)  [unwired: 5 in]
        n47 = case shown="False" w110 {
          tunnel: w109 -> [w114 w116]
          tunnel: [w114 w115] -> w108
          frame False {
            # "Do not stop testing"
          }
          frame True {
            # "Stop Testing"
            n48 = property on="Start" class="Bool (strict)"(error in=w116, "Val(Sgnl)"=FALSE ("Value (Signaling)")) -> (error out=w115:errorcluster)  [unwired: 1 in, 1 out]
          }
        }
      }
      frame "Reset Device" {
        n49 = call "Reset DUT.vi"("error in (no error)"=w120, "State-machine Local Variables in"=w122) -> ("error out"=w119:errorcluster, "State-machine Local Variables out"=w118:T6)  [unwired: 8 in]
      }
      frame "Scan Channels" {
        # "Scans all channels for a transmitting device. \nWill display results to Message board."
        n50 = control-ref of="This VI"() -> (w123:refnum<vi>)
        n51 = call "Scan All Channels.vi"("error in (no error)"=w128, "VI in"=w123, "State-machine Local Variables in"=w124) -> ("error out"=w127:errorcluster, "State-machine Local Variables out"=w126:T6)  [unwired: 7 in]
      }
      frame "Shutdown Device" {
        w137 = FALSE  # Blast?
        n52 = local read "Device ON?"() -> (w134:bool)
        n53 = call "Shutdown DUT.vi"("error in (no error)"=w135, "Device On?"=w134, "Blast?"=w137, "Data In"=w136) -> ("error out"=w131:errorcluster, "State-machine Local Variables out"=w132:T6)  [unwired: 6 in]
        n54 = call "RxBuffer.vi"("Clear?"=TRUE, "error in (no error)"=w131) -> ("error out"=w130:errorcluster)  [unwired: 6 in, 11 out]
      }
      frame "Timeout", Default {
        n55 = event shown="[3] \"A2 Delay (ms)\": Value Change" {
          selector: _ -> [_ _ _ _ _ _ _ _ _ _ _ _ _ _ _ _ _ _ _ _ _ _ _ _ _]
          dyn-events: _ -> [_ _ _ _ _ _ _ _ _ _ _ _ _ _ _ _ _ _ _ _ _ _ _ _ _]
          timeout: 5 -> [_ _ _ _ _ _ _ _ _ _ _ _ _ _ _ _ _ _ _ _ _ _ _ _ _]
          tunnel: [w150 Gen2_FT_states."Timeout" ("Current State Out") Gen2_FT_states."Timeout" ("Current State Out") Gen2_FT_states."Timeout" ("Current State Out") Gen2_FT_states."Timeout" ("Current State Out") Gen2_FT_states."Timeout" ("Current State Out") Gen2_FT_states."Exit" ("Current State Out") w287 Gen2_FT_states."Timeout" ("Current State Out") Gen2_FT_states."Timeout" ("Current State Out") Gen2_FT_states."Timeout" ("Current State Out") Gen2_FT_states."Timeout" ("Current State Out") Gen2_FT_states."Timeout" ("Current State Out") Gen2_FT_states."Timeout" ("Current State Out") Gen2_FT_states."Timeout" ("f") Gen2_FT_states."Timeout" ("Current State Out") Gen2_FT_states."Timeout" ("Current State Out") Gen2_FT_states."Timeout" ("Current State Out") Gen2_FT_states."Timeout" ("Current State Out") Gen2_FT_states."Timeout" ("Current State Out") Gen2_FT_states."Initialization" ("Current State Out") Gen2_FT_states."Timeout" ("Current State Out") Gen2_FT_states."Timeout" ("Current State Out") Gen2_FT_states."Timeout" ("Current State Out") Gen2_FT_states."Timeout" ("Current State Out")] -> w144
          tunnel: w143 -> [w149 w192 w197 w202 w209 w282 w285 w291 w293 w324 w329 w341 w347 w355 w371 w464 w468 w475 w487 w493 w496 w521 w552 w567 w576]
          tunnel: [w151 w189 w194 w200 w208 w281 w285 w291 w300 w322 w327 w335 w344 w354 w370 w464 w467 w473 w486 w491 w495 w510 w551 w562 w571] -> w138
          tunnel: w142 -> [w152 _ _ _ _ _ _ _ _ _ _ _ _ _ _ _ _ _ _ _ _ _ _ _ _]
          tunnel: w141 -> [w148 _ _ _ _ _ _ w288 _ _ _ _ _ _ w369 _ _ _ _ _ _ _ _ _ _]
          tunnel: w140 -> [w147 w191 w196 w201 w204 w280 w284 w290 w292 w323 w328 w337 w346 w348 w367 w465 w470 w474 w477 w492 w498 w512 w555 w565 w573]
          tunnel: [w147 w191 w196 w201 w204 w280 w284 w290 w295 w323 w328 w336 w346 w348 w366 w465 w470 w474 w476 w492 w498 w512 w554 w564 w573] -> w139
          event Timeout {
            n56 = event-data() -> ()  [unwired: 1 in, 1 out]
            n57 = case shown="False" w148 {
              tunnel: w152 -> [w171 _]
              tunnel: [w163 w186] -> w151
              tunnel: [w162 Gen2_FT_states."Timeout" ("NextState")] -> w150
              tunnel: w149 -> [w156 w186]
              frame False {
                n58 = Quotient & Remainder(x=w171, y=5) -> (x-y*floor(x/y)=w169:i32)  [unwired: 1 out]
                n59 = Unbundle By Name(w156) -> ("Scroll Message?"=w157:bool, "NextState"=w168:T4, "Target Information.Target DevID"=→"DeviceID:":u32, "PCB Score"=→"PCB Score":i32, "AssyScore"=→"AssemScore":i32, "Channels.Transceiver Ch"=→"Transceiver Channel:":u8)
                n60 = Equal To 0?(x=w169) -> (x = 0?=w167:bool)
                n61 = call "MessageHandler.vi"("State-machine Local Variables"=w156) -> ("Message Out"=→"Message":string, "State-machine Local Variables out"=w155:T6)  [unwired: 7 in]
                n62 = case shown="True" w157 {
                  frame False {
                  }
                  frame True {
                    n63 = property on="Message" class="Str"("Text.Scroll Position"=u32 10000) -> ()  [unwired: 2 in, 2 out]
                  }
                }
                n64 = case shown="Default" w168 {
                  selector: w168 -> [w179 w182]
                  tunnel: [w179 w183] -> w162
                  tunnel: w167 -> [_ w184]
                  tunnel: w155 -> [w178 w181]
                  tunnel: [w178 w181] -> w158
                  frame Default {
                  }
                  frame "Timeout" {
                    n65 = Select(t=Gen2_FT_states."Display Result" ("Current State Out"), s=w184, f=w182) -> (s? t:f=w183:T4)
                  }
                }
                n66 = Unbundle By Name(w158) -> ("ScanTime"=w165:timestamp)
                n67 = Get Date/Time In Seconds() -> (seconds since 1Jan1904=w166:timestamp)
                n68 = Greater?(x=w166, y=w165) -> (0:w164:bool)
                n69 = case shown="True" w164 {
                  tunnel: w158 -> [w173 w177]
                  tunnel: [w173 w176] -> w163
                  frame False {
                  }
                  frame True {
                    n70 = Bundle By Name(cluster=w177, "Valid String?"=FALSE, "ScannedString"="") -> (w176:T6)
                  }
                }
              }
              frame True {
                n71 = local write "Message"("EMERGENCY STOP BUTTON IS ENABLED..." ("Message")) -> ()
              }
            }
          }
          event "Message": Mouse Enter {
            n72 = event-data() -> ()  [unwired: 1 in, 4 out]
            n73 = Bundle By Name(cluster=w192, "Scroll Message?"=FALSE ("Stop Scroll?")) -> (w189:T6)
          }
          event "Message": Mouse Leave {
            n74 = event-data() -> ()  [unwired: 1 in, 4 out]
            n75 = Bundle By Name(cluster=w197, "Scroll Message?"=TRUE ("Scroll?")) -> (w194:T6)
          }
          event "A2 Delay (ms)": Value Change {
            n76 = event-data() -> ()  [unwired: 1 in, 6 out]
            n77 = Bundle By Name(cluster=w202, "A2 Delay (msec)"="A2 Delay (ms)") -> (w200:T6)
          }
          event Key Down {
            w211 = i16 37  # ScanCode for "k"
            n78 = event-data() -> ("ScanCode"=w206:i16, "PlatMods"=w212:T23, "Char"=w207:i16)  [unwired: 1 in]
            n79 = Equal?(x=w211, y=w206) -> (x = y?=w213:bool)
            n80 = Unbundle By Name(w212) -> ("Ctrl"=w205:bool)
            n81 = And(x=w213, y=w205) -> (x .and. y?=w210:bool)
            n82 = case shown="False" w210 {
              tunnel: w209 -> [w216 w265]
              tunnel: [w215 w265] -> w208
              tunnel: w207 -> [w214 _]
              frame False {
                n83 = Unbundle By Name(w216) -> ("Valid String?"=w217:bool)
                n84 = case shown="False" w217 {
                  tunnel: w216 -> [w243 w263]
                  tunnel: [w218 w263] -> w215
                  tunnel: w214 -> [w226 _]
                  frame False {
                    (unwired) "\n"
                    n85 = Unbundle By Name(w243) -> ("ScanTime"=w233:timestamp, "ScannedString"=w242:string)
                    n86 = Get Date/Time In Seconds() -> (seconds since 1Jan1904=w225:timestamp)
                    n87 = case shown="\"\"" w242 {
                      selector: w242 -> [w254 w258]
                      tunnel: [w256 w261] -> w241
                      tunnel: w243 -> [w256 w262]
                      tunnel: w233 -> [w255 _]
                      tunnel: [w255 w259] -> w232
                      tunnel: [w254 w258] -> w231
                      tunnel: w225 -> [_ w257]
                      frame Default {
                      }
                      frame "" {
                        w260 = 5.0  # Allowed ScanTime (Sec)
                        # "Starting of string,\nso start timer"
                        n88 = Add(x=w257, y=w260) -> (x+y=w259:timestamp)
                        n89 = Bundle By Name(cluster=w262, "ScanTime"=w259) -> (w261:T6)
                      }
                    }
                    n90 = Type Cast(type="", x=w226) -> (*(type *) &x=w236:string)
                    n91 = Reverse String(1:w236) -> (0:w237:string)
                    n92 = String Subset(string=w237, length (rest)=1 ("length (rest)")) -> (substring=w230:string)  [unwired: 1 out]
                    n93 = case shown="Default" w230 {
                      selector: w230 -> [w245 _]
                      tunnel: [w245 _] -> w229
                      tunnel: [_ w246] -> w223
                      tunnel: w226 -> [_ w247]
                      frame ",", "-", ".", "/", "0", "1", "2", "3", "4", "5", "6", "7", "8", "9", ":", "A".."Z", "[", "]", "a".."z" {
                      }
                      frame Default {
                        n94 = Equal To 0?(x=w247) -> (x = 0?=w246:bool)
                      }
                    }
                    n95 = Greater?(x=w225, y=w232) -> (0:w224:bool)
                    n96 = Concatenate Strings(w231, w229) -> (w244:string)
                    n97 = call "BatchTest BoolValue Change.vi"("Value In"=w223) -> ("Value Changed?"=w221:bool, "Value Out"=w222:bool)  [unwired: 7 in, 2 out]
                    n98 = And(x=w222, y=w221) -> (x .and. y?=w220:bool)
                    n99 = Select(t="", s=w224, f=w244) -> (s? t:f=w228:string)
                    n100 = call "ValidateScan.vi"("LF?"=w220, "String In"=w228) -> ("Valid Format?"=w227:bool, "ScanData"=w234:T24, "String Out"=w235:string)  [unwired: 6 in, 1 out]
                    n101 = Bundle By Name(cluster=w241, "ScannedString"=w235, "Valid String?"=w227) -> (w219:T6)
                    n102 = case shown="True" w227 {
                      tunnel: w234 -> [_ w253]
                      tunnel: w219 -> [w248 w252]
                      tunnel: [w248 w251] -> w218
                      frame False {
                      }
                      frame True {
                        n103 = Unbundle By Name(w253) -> ("DeviceID"=w250:u32, "Mfg Date"=w249:timestamp)
                        n104 = Bundle By Name(cluster=w252, "LabelDevID"=w250, "MfgDate"=w249) -> (w251:T6)
                      }
                    }
                  }
                  frame True {
                  }
                }
              }
              frame True {
                # "1350x681  or   937x681  for HP Laptop"
                n105 = control-ref of="This VI"() -> (w271:refnum<vi>)
                n106 = property class="VI"(reference=w271) -> (reference out=w273:refnum<vi>, "Front Panel.PanelBounds"=w272:T25)  [unwired: 1 in, 1 out]
                n107 = Unbundle By Name(w272) -> ("Right"=w270:i16, "Left"=w268:i16)
                n108 = Subtract(x=w270, y=w268) -> (x-y=w269:i16)
                n109 = case shown="937" w269 {
                  tunnel: [i16 937 i16 1350] -> w267
                  frame Default {
                  }
                  frame 937 {
                  }
                }
                n110 = Add(x=w267, y=w268) -> (x+y=w266:i16)
                n111 = Bundle By Name(cluster=w272, "Right"=w266) -> (w264:T25)
                n112 = property class="VI"(reference=w273, "Front Panel.PanelBounds"=w264) -> ()  [unwired: 1 in, 2 out]
              }
            }
          }
          event "Shutdown Dev": Value Change {
            n113 = event-data() -> ()  [unwired: 1 in, 5 out]
            n114 = Bundle By Name(cluster=w282, "Message"="Attempting to turn OFF the Device, please wait...", "Shutdown Counter"=u32 0, "NextState"=Gen2_FT_states."Shutdown Device" ("Current State Out")) -> (w281:T6)
          }
          event "Exit": Value Change {
            n115 = event-data() -> ()  [unwired: 1 in, 5 out]
          }
          event Value Change {
            n116 = event-data() -> ()  [unwired: 1 in, 5 out]
            n117 = Select(t=Gen2_FT_states."ESTOP" ("Current State Out"), s=w288, f=Gen2_FT_states."Timeout") -> (s? t:f=w287:T4)
          }
          event "Device ON?": Value Change {
            n118 = event-data() -> ("NewVal"=w299:bool)  [unwired: 1 in]
            n119 = First Call?() -> (First Call?: T/F=w297:bool)
            n120 = Not(x=w297) -> (.not. x?=w296:bool)
            n121 = And(x=w296, y=w299) -> (x .and. y?=w298:bool)
            n122 = case shown="True" w298 {
              tunnel: w293 -> [w306 w310]
              tunnel: [w305 w314] -> w300
              tunnel: w292 -> [w303 w312]
              tunnel: [w301 w308] -> w295
              frame False {
                n123 = call "RxBuffer.vi"("Clear?"=TRUE, "error in (no error)"=w303) -> ("error out"=w301:errorcluster)  [unwired: 6 in, 11 out]
                n124 = Bundle By Name(cluster=w306, "RXTX Window Found?"=FALSE) -> (w305:T6)
              }
              frame True {
                n125 = call "RxBuffer.vi"("error in (no error)"=w312) -> ("DeviceParameters"=w311:T26, "error out"=w308:errorcluster)  [unwired: 7 in, 10 out]
                n126 = call "Device On.vi"("DeviceParameters"=w311, "Data In"=w310) -> ("Data Out"=w307:T6)  [unwired: 9 in]
                n127 = Unbundle By Name(w307) -> ("DUT Parameters"=→"Device Parameters":T2, "RXTX Window Found?"=w313:bool)
                n128 = case shown="False" w313 {
                  tunnel: [w318 w319] -> w314
                  tunnel: w307 -> [w315 w319]
                  frame False {
                    n129 = Bundle By Name(cluster=w315, "Message"="Attempting to Find RxTx Window. Please wait this could take up to 30 seconds", "NextState"=Gen2_FT_states."Find RxTx Window") -> (w318:T6)
                  }
                  frame True {
                    # "Window has already been found. No need to find it again"
                  }
                }
              }
            }
          }
          event "Operator": Value Change {
            n130 = event-data() -> ()  [unwired: 1 in, 6 out]
            n131 = Bundle By Name(cluster=w324, "Operator"="Operator") -> (w322:T6)
          }
          event Value Change {
            n132 = event-data() -> ()  [unwired: 1 in, 6 out]
            n133 = Bundle By Name(cluster=w329, "DUT Parameters.Lot#"="Lot#:") -> (w327:T6)
          }
          event "Start Channel:": Value Change {
            w338 = TRUE ("RF Chip0 Enable")
            w339 = XceiverCmds."Set Channel" ("XceiverCmd")
            # "Change RF Channel"
            n134 = event-data() -> ()  [unwired: 1 in, 6 out]
            n135 = Decimal String To Number(string="Start Channel:") -> (number=w330:i32)  [unwired: 2 in, 1 out]
            n136 = call "XceiverCmds.vi"("RF Chip0 Channel"=w330, "RF Chip1 Channel"=w330, "error in (no error)"=w337, "XceiverCmd"=w339) -> ("error out"=w340:errorcluster)  [unwired: 9 in, 2 out]
            n137 = call "XceiverCmds.vi"("RF Chip0 Channel"=w330, "RF Chip0 Enable"=w338, "RF Chip1 Enable"=w338, "RF Chip1 Channel"=w330, "error in (no error)"=w340, "XceiverCmd"=w339) -> ("error out"=w336:errorcluster)  [unwired: 7 in, 2 out]
            n138 = Concatenate Strings("RF Channel Changed to: ", "Start Channel:") -> (w333:string)
            n139 = Bundle By Name(cluster=w341, "Channels.Transceiver Ch"=w330, "Message"=w333, "Channels.Start Ch"=w330) -> (w335:T6)
          }
          event Value Change {
            n140 = event-data() -> ()  [unwired: 1 in, 6 out]
            n141 = Decimal String To Number(string="Target Channel:") -> (number=w342:i32)  [unwired: 2 in, 1 out]
            n142 = Bundle By Name(cluster=w347, "Target Information.Target Channel"=w342) -> (w344:T6)
          }
          event "Reset Device": Value Change {
            n143 = event-data() -> ()  [unwired: 1 in, 6 out]
            n144 = disable-structure shown="Enabled" {
              disable-tunnel: [w362 w364] -> w353
              disable-tunnel: "Attempting to reset device" -> [w361 w364]
              disable-tunnel: Gen2_FT_states."Reset Device" ("NextState") -> [w359 w363]
              disable-tunnel: [w357 w363] -> w349
              frame Disabled {
                n145 = local read "Device ON?"() -> (w356:bool)
                n146 = Select(t=w361, s=w356, f="No Device Detected") -> (s? t:f=w362:string)
                n147 = Select(t=w359, s=w356, f=Gen2_FT_states."Timeout") -> (s? t:f=w357:T4)
              }
              frame Enabled {
              }
            }
            n148 = Bundle By Name(cluster=w355, "Message"=w353, "NextState"=w349) -> (w354:T6)
          }
          event "Start": Value Change {
            n149 = event-data() -> ("NewVal"=w372:bool)  [unwired: 1 in]
            n150 = case shown="True" w372 {
              tunnel: w371 -> [w375 w391]
              tunnel: [w387 w397] -> w370
              tunnel: w369 -> [_ w396]
              tunnel: w367 -> [w374 w392]
              tunnel: [w376 w392] -> w366
              frame False {
                w377 = TRUE ("RF Chip0 Enable")
                w383 = XceiverCmds."Set Channel" ("XceiverCmd")
                n151 = Unbundle By Name(w375) -> ("Channels.Start Ch"=w373:u8)
                n152 = call "XceiverCmds.vi"("RF Chip0 Channel"=w373, "RF Chip1 Channel"=w373, "error in (no error)"=w374, "XceiverCmd"=w383) -> ("error out"=w384:errorcluster)  [unwired: 9 in, 2 out]
                n153 = call "XceiverCmds.vi"("RF Chip0 Channel"=w373, "RF Chip0 Enable"=w377, "RF Chip1 Enable"=w377, "RF Chip1 Channel"=w373, "error in (no error)"=w384, "XceiverCmd"=w383) -> ("error out"=w376:errorcluster)  [unwired: 7 in, 2 out]
                n154 = Bundle By Name(cluster=w375, "Message"="Testing was stopped.", "NextState"=Gen2_FT_states."End Test" ("Current State Out"), "Test Result"=FALSE ("Result"), "Result String"="Testing Stopped.", "Channels.Transceiver Ch"=w373) -> (w387:T6)
                n155 = local write "BatteryCapState"(i8 0 ("BatteryCapState")) -> ()
                n156 = property on="CaptureButton" class="Bool (strict)"("Visible"=FALSE) -> ()  [unwired: 2 in, 2 out]
                n157 = global write "Gen2 FT Globals.vi" "RawRxTx"(FALSE ("RawRxTx")) -> ()
              }
              frame True {
                n158 = Unbundle By Name(w391) -> ("Operator"=w390:string, "Eng-Result#"=w389:u32, "Channels.Transceiver Ch"=w388:u8)
                n159 = Empty String/Path?(string/path=w390) -> (empty?=w398:bool)
                n160 = Equal To 0?(x=w389) -> (x = 0?=w393:bool)
                n161 = Compound Arithmetic op=OR(w396, w398, w393) -> (w395:T3)
                n162 = Not(x=w395) -> (.not. x?=w394:T3)
                n163 = case shown="True" w394 {
                  tunnel: w391 -> [w417 w422]
                  tunnel: [w405 w423] -> w397
                  tunnel: w396 -> [_ _]
                  tunnel: w398 -> [w404 _]
                  tunnel: w393 -> [w402 _]
                  tunnel: w389 -> [_ w420]
                  tunnel: w388 -> [_ w421]
                  frame False {
                    w401 = FALSE ("s")
                    n164 = Select(t="Please enter an Operator name...", s=w404, f="") -> (s? t:f=w406:string)
                    n165 = Select(t="Please enter a Eng-Result#        \n", s=w402, f=w406) -> (s? t:f=w407:string)
                    n166 = local write "Start"(FALSE ("Start")) -> ()
                    n167 = Select(t="Please enter a valid Lot number...", s=w401, f=w407) -> (s? t:f=w399:string)
                    n168 = Select(t="Please select a DeviceType...", s=w401, f=w399) -> (s? t:f=w408:string)
                    n169 = Select(t="Please select a device Brand...", s=w401, f=w408) -> (s? t:f=w409:string)
                    n170 = Select(t="Please release E-Stop...", s=w401, f=w409) -> (s? t:f=w415:string)
                    n171 = Bundle By Name(cluster=w417, "Message"=w415) -> (w405:T6)
                  }
                  frame True {
                    n172 = property on="Shutdown Dev" class="Bool"("DisabledEnum"=T19."Disabled" ("Disabled")) -> ()  [unwired: 2 in, 2 out]
                    n173 = case shown="Default" w421 {
                      tunnel: w422 -> [w429 w441]
                      tunnel: [w436 w442] -> w423
                      tunnel: w420 -> [w424 w439]
                      frame 3 {
                        w433 = u32 13466634  # Serial Number
                        # "Blank Device"
                        n174 = call "FindEEPROMandInputScriptPathandLetter.vi"("Eng-Result #"=w424, "Create New Engr Results? (F)"=TRUE ("Create Eng Results File?")) -> ()  [unwired: 5 in, 3 out]
                        n175 = Unbundle By Name(w429) -> ("Support Script.Default GAINC"=w428:string)
                        n176 = Random Number (0-1)() -> (number: 0 to 1=w430:dbl)
                        n177 = Multiply(x=w430, y=10000.0) -> (x*y=w427:dbl)
                        n178 = Bundle By Name(cluster=w429, "Message"="Attempting to locate Blank Device and program it...This may take a few minutes", "DUT Serial #"=w433, "Programming Step"=Iniial_Device_Programming."Load EEPROM", "Final Program?"=FALSE ("Blank Device?"), "GAINC Value"=w428, "Programming Mode"=ProgramStageControl."Initial Program" ("Program Stage"), "Batt Test Step"=Batt_Cap_Steps."Initialize" ("Batt Capture State"), "Target Information.Target Serial#"=w427, "NextState"=Gen2_FT_states."Program Device" ("Current State Out")) -> (w436:T6)
                      }
                      frame Default {
                        # "Channels 2, 4,5,6,7"
                        n179 = local read "Device ON?"() -> (w440:bool)
                        n180 = case shown="False" w440 {
                          tunnel: [w448 w460] -> w442
                          tunnel: w441 -> [w447 w458]
                          tunnel: w439 -> [_ w450]
                          frame False {
                            w443 = T19."Enabled" ("Disabled")
                            n181 = local write "Start"(FALSE ("Start")) -> ()
                            n182 = property on="Shutdown Dev" class="Bool"("DisabledEnum"=w443) -> ()  [unwired: 2 in, 2 out]
                            n183 = property on="Start Channel:" class="CmbBox"("DisabledEnum"=w443) -> ()  [unwired: 2 in, 2 out]
                            n184 = Bundle By Name(cluster=w447, "Message"="No Device detected.", "NextState"=Gen2_FT_states."Timeout") -> (w448:T6)
                          }
                          frame True {
                            n185 = call "FindEEPROMandInputScriptPathandLetter.vi"("Eng-Result #"=w450, "Create New Engr Results? (F)"=TRUE) -> ()  [unwired: 5 in, 3 out]
                            n186 = Random Number (0-1)() -> (number: 0 to 1=w453:dbl)
                            n187 = Multiply(x=w453, y=10000.0) -> (x*y=w452:dbl)
                            n188 = Bundle By Name(cluster=w458, "Target Information.Target Serial#"=w452, "Programming Step"=Iniial_Device_Programming."Load EEPROM", "Programming Mode"=ProgramStageControl."Scales" ("Program Stage"), "Batt Test Step"=Batt_Cap_Steps."Initialize" ("Batt Capture State"), "Final Program?"=TRUE ("Blank Device?"), "NextState"=Gen2_FT_states."Battery Test" ("f")) -> (w460:T6)
                          }
                        }
                      }
                    }
                    n189 = property on="Start Channel:" class="CmbBox"("DisabledEnum"=T19."Disabled and Grayed Out" ("Disabled")) -> ()  [unwired: 2 in, 2 out]
                  }
                }
              }
            }
            n190 = property on="Test Result" class="Bool (strict)"("Colors [4]"=cluster{u32, u32}[] [{12369084, 12369084}, {12369084, 12369084}, {1985280, 1985280}, {1985280, 1985280}]) -> ()  [unwired: 2 in, 2 out]
          }
          event "Save EEPROM Data": Value Change {
            n191 = event-data() -> ()  [unwired: 1 in, 2 out]
            n192 = Unbundle By Name(w464) -> ("EEPROM Data"=w463:i32[][])
            n193 = call-poly <vilib>:"Write To Spreadsheet File.vi"("delimiter (\\t)"="," ("delimiter (\\t)"), "2D data"=w463) -> ()  [unwired: 6 in, 1 out]
          }
          event "Clear Message": Value Change {
            n194 = event-data() -> ()  [unwired: 1 in, 2 out]
            n195 = Bundle By Name(cluster=w468, "Clear Message"=TRUE) -> (w467:T6)
          }
          event "Eng-Result# :": Value Change {
            n196 = event-data() -> ()  [unwired: 1 in, 2 out]
            n197 = Bundle By Name(cluster=w475, "Eng-Result#"="Eng-Result# :") -> (w473:T6)
          }
          event "CaptureButton": Value Change {
            n198 = event-data() -> ()  [unwired: 1 in, 6 out]
            n199 = Unbundle By Name(w487) -> ("Batt Test Step"=w481:T9)
            n200 = property on="CaptureButton" class="Bool (strict)"(error in=w477, "Visible"=FALSE, "DisabledEnum"=T19."Disabled" ("Disabled"), "Value"=FALSE ("CaptureButton")) -> (error out=w476:errorcluster)  [unwired: 1 in, 1 out]
            n201 = Increment(x=w481) -> (x+1=w479:T9)
            n202 = Bundle By Name(cluster=w487, "Batt Test Step"=w479, "NextState"=Gen2_FT_states."Battery Test", "Message"="Collecting Voltage....") -> (w486:T6)
          }
          event "Scan Channels": Value Change {
            n203 = event-data() -> ()  [unwired: 1 in, 6 out]
            n204 = Bundle By Name(cluster=w493, "Message"="Scanning for Devices. Please Wait.", "NextState"=Gen2_FT_states."Scan Channels") -> (w491:T6)
          }
          event "Mark-10 COM Port": Value Change {
            n205 = event-data() -> ()  [unwired: 1 in, 6 out]
            n206 = call <vilib>:"Application Directory.vi"() -> ("Application Directory"=w506:path)
            n207 = Bundle By Name(cluster=w496, "COM Port"="Mark-10 COM Port") -> (w495:T6)
            n208 = Build Path(base path=w506, name or relative path=path "Mark-10ComPort.ini") -> (appended path=w504:path)
            n209 = call <vilib>:"Open Config Data.vi"("configuration file path"=w504) -> ("refnum"=w503:T27)  [unwired: 8 in, 2 out]
            n210 = call-poly <vilib>:"Write Key.vi"("section"="Mark-10 Com Port", "value"="Mark-10 COM Port", "key"="Com", "refnum"=w503) -> ("error out"=w499:errorcluster, "refnum out"=w500:T27)  [unwired: 5 in, 1 out]
            n211 = call <vilib>:"Close Config Data.vi"("error in (no error)"=w499, "refnum"=w500) -> ()  [unwired: 8 in, 2 out]
            n212 = call "Mark10.vi"("Data In"=w495, "Action"=Mark10_states."Initialize") -> ()  [unwired: 13 in, 5 out]
          }
          event "Brand:": Value Change {
            n213 = event-data() -> ("NewVal"=w508:string)  [unwired: 1 in]
            n214 = property on="Brand:" class="CmbBox"() -> ("Strings[]"=w528:string[])  [unwired: 2 in, 2 out]
            n215 = Unbundle By Name(w521) -> ("PendingDeviceType"=w524:string, "Support Script.[[DeviceTypes]]"=w527:string[][])
            n216 = Search 1D Array(1D array=w528, element=w508) -> (index of element=w526:i32)  [unwired: 1 in]
            n217 = Decrement(x=w526) -> (x-1=w516:i32)
            n218 = Index Array(array=w527, index (row)=w516) -> (element=w518:string[])  [unwired: 1 in]
            n219 = Index Array(array=w518) -> (element=w522:string)  [unwired: 1 in]
            n220 = Search 1D Array(1D array=w518, element="", start index (0)=1) -> (index of element=w517:i32)
            n221 = case shown="\"\"" w524 {
              selector: w524 -> [w542 _]
              tunnel: [w542 w543] -> w523
              tunnel: w522 -> [_ w543]
              frame Default {
              }
              frame "" {
              }
            }
            n222 = case shown="-1" w517 {
              selector: w517 -> [w533 _]
              tunnel: [w535 w536] -> w525
              tunnel: w518 -> [w534 w536]
              frame Default {
                n223 = Array Subset(array=w534, length=w533) -> (w535:string[])  [unwired: 1 in]
              }
              frame -1 {
              }
            }
            n224 = flat-sequence {
              tunnel: w525 -> [w538]
              tunnel: w523 -> [w537]
              tunnel: w521 -> [w541]
              tunnel: [w540] -> w514
              frame #0 {
                n225 = property on="DeviceType:" class="CmbBox"("Strings[]"=w538, "Value"=w537) -> ()  [unwired: 2 in, 2 out]
              }
              frame #1 {
                n226 = Bundle By Name(cluster=w541, "PendingDeviceType"="") -> (w540:T6)
              }
            }
            n227 = Empty String/Path?(string/path=w508) -> (empty?=w515:bool)
            n228 = case shown="True" w515 {
              tunnel: w514 -> [w529 w532]
              tunnel: [w529 w531] -> w513
              frame False {
              }
              frame True {
                n229 = Bundle By Name(cluster=w532, "Target Information.Target DevID"=u32 0 ("DeviceID:")) -> (w531:T6)
              }
            }
            n230 = Bundle By Name(cluster=w513, "DUT Parameters.Brand"="Brand:") -> (w510:T6)
          }
          event "Get Window": Value Change {
            n231 = event-data() -> ()  [unwired: 1 in, 6 out]
            n232 = call "XceiverCmds.vi"("error in (no error)"=w555, "XceiverCmd"=XceiverCmds."Get Window") -> ("unsigned byte array"=w550:u8[], "error out"=w554:errorcluster)  [unwired: 11 in, 1 out]
            n233 = Index Array(array=w550, index=1) -> (element=w549:u8)
            n234 = Number To Decimal String(number=w549) -> (decimal integer string=w546:string)  [unwired: 1 in]
            n235 = Concatenate Strings("Window Found: " ("string"), w546, " msecs" ("string")) -> (w548:string)
            n236 = Bundle By Name(cluster=w552, "Message"=w548) -> (w551:T6)
          }
          event "Set Wndow": Value Change {
            n237 = event-data() -> ()  [unwired: 1 in, 6 out]
            n238 = call "XceiverCmds.vi"("mSec"="mSec", "error in (no error)"=w565, "XceiverCmd"=XceiverCmds."Set Window") -> ("error out"=w564:errorcluster)  [unwired: 10 in, 2 out]
            n239 = Number To Decimal String(number="mSec") -> (decimal integer string=w559:string)  [unwired: 1 in]
            n240 = Concatenate Strings("RxTX Window Set: ", w559, " msecs" ("string")) -> (w557:string)
            n241 = Bundle By Name(cluster=w567, "Message"=w557) -> (w562:T6)
          }
          event "DeviceType:": Value Change {
            n242 = event-data() -> ("NewVal"=w569:string)  [unwired: 1 in]
            n243 = Unbundle By Name(w576) -> ("DUT Parameters.Brand"=w568:string, "Target Information.Target DevID"=w575:u32)
            n244 = case shown="Default" w569 {
              selector: w569 -> [_ w590]
              tunnel: w576 -> [_ w587]
              tunnel: [w585 w589] -> w577
              tunnel: w575 -> [w585 w588]
              tunnel: w568 -> [_ w586]
              frame "" {
              }
              frame Default {
                n245 = case shown="Default" w586 {
                  selector: w586 -> [_ w600]
                  tunnel: w590 -> [_ w603]
                  tunnel: w587 -> [_ w599]
                  tunnel: [w591 w596] -> w589
                  tunnel: w588 -> [w591 _]
                  tunnel: w587 -> [_ _]
                  frame "" {
                  }
                  frame Default {
                    n246 = property on="DeviceType:" class="CmbBox"() -> ("Strings[]"=w604:string[])  [unwired: 2 in, 2 out]
                    n247 = property on="Brand:" class="CmbBox"() -> ("Strings[]"=w601:string[])  [unwired: 2 in, 2 out]
                    n248 = Search 1D Array(1D array=w601, element=w600, start index (0)=1) -> (index of element=w595:i32)
                    n249 = Search 1D Array(1D array=w604, element=w603, start index (0)=1) -> (index of element=w593:i32)
                    n250 = Unbundle By Name(w599) -> ("Support Script.[[DeviceTypesVals]]"=w598:u16[][])
                    n251 = Decrement(x=w595) -> (x-1=w594:i32)
                    n252 = Decrement(x=w593) -> (x-1=w592:i32)
                    n253 = Index Array(array=w598, index (row)=w594, index (col)=w592) -> (element=w596:u16)
                    n254 = property on="DeviceID:" class="DigNum (strict)"("Value"=w596) -> ()  [unwired: 2 in, 2 out]
                  }
                }
              }
            }
            n255 = Empty String/Path?(string/path=w569) -> (empty?=w574:bool)
            n256 = case shown="True" w574 {
              tunnel: [w581 w584] -> w578
              tunnel: w577 -> [w580 _]
              tunnel: w576 -> [w579 w583]
              frame False {
                n257 = Bundle By Name(cluster=w579, "Target Information.Target DevID"=w580) -> (w581:T6)
              }
              frame True {
                n258 = Bundle By Name(cluster=w583, "Target Information.Target DevID"=u32 0 ("DevID")) -> (w584:T6)
              }
            }
            n259 = Bundle By Name(cluster=w578, "Target Information.Target DeviceType"="DeviceType:") -> (w571:T6)
          }
        }
        n260 = Get Date/Time In Seconds() -> (seconds since 1Jan1904=→"Current Time:":timestamp)
      }
      frame "Program Device" {
        n261 = call "Program Device Main.vi"("error in (no error)"=w609, "Data In"=w606) -> ("error out"=w608:errorcluster, "Data Out"=w605:T6)  [unwired: 8 in]
        n262 = Unbundle By Name(w605) -> ("EEPROM Data"=→"EEPROM Data":i32[][])
      }
      frame "Battery Test" {
        # "1. Collect battery voltage for 10 seconds \n\n2. Store data in support file\n\n3. Move to program the device end test."
        n263 = Unbundle By Name(w614) -> ("Batt Test Step"=w613:T9)
        n264 = case shown="\"Check Results\"" w613 {
          tunnel: w614 -> [w627 w639 w659 w681]
          tunnel: [w626 w637 w657 w684] -> w615
          tunnel: w612 -> [w623 w633 w653 w670]
          tunnel: [w621 w632 w653 w669] -> w611
          frame "Initialize", Default {
            w619 = dbl[][] [] ("[A/Ds]")
            # "Pulls the Zero Load A/D counts which is saved when Batt Collection\nis complete."
            # "Tell the operator to set the Power supply to 2.80 volts"
            n265 = property on="CaptureButton" class="Bool (strict)"(error in=w623, "Visible"=TRUE, "DisabledEnum"=T19."Enabled" ("Disabled"), "Value"=FALSE) -> (error out=w622:errorcluster)  [unwired: 1 in, 1 out]
            n266 = Bundle By Name(cluster=w627, "[A/Ds]"=w619) -> (w620:T6)
            n267 = call "RxBuffer.vi"("error in (no error)"=w622) -> ("LoadSensors"=w618:dbl[], "error out"=w621:errorcluster)  [unwired: 7 in, 10 out]
            n268 = Build Array (concatenate)(w619, w618) -> (w617:dbl[][])
            n269 = Bundle By Name(cluster=w620, "Message"="Adjust the Power Supply to 2.80 volts. When ready click the capture button...", "NextState"=Gen2_FT_states."Timeout", "[A/Ds]"=w617) -> (w626:T6)
          }
          frame "Collect 2.8 Volts" {
            # "Average the 50 \nBattery readings"
            # "2.80V"
            # "Collect the Battery readings that correspond to 2.80 volts.\nCollct them for 5 seconds."
            n270 = for {
              N: 50 -> [_]
              shift-right: [w646] -> w640
              shift-left: u64 0 -> [w648]
              tunnel: [TRUE ("Visible")] -> w634
              # "Add all the Battery readings, \nso that an average can be \ncalculated later."
              # "Pull out the Battery reading from\neach set of data."
              n271 = call "RxBuffer.vi"() -> ("RxData Out"=w650:u16[])  [unwired: 8 in, 11 out]
              n272 = Wait (ms)(milliseconds to wait=u32 100) -> ()  [unwired: 1 out]
              n273 = Index Array(array=w650, index=10) -> (element=w647:u16)
              n274 = Add(x=w647, y=w648) -> (x+y=w646:u64)
            }
            n275 = Divide(x=w640, y=u64 50) -> (x/y=w631:dbl)
            "Batt280" <- w631
            n276 = property on="CaptureButton" class="Bool (strict)"(error in=w633, "Visible"=w634, "DisabledEnum"=T19."Enabled" ("Disabled"), "Value"=FALSE) -> (error out=w632:errorcluster)  [unwired: 1 in, 1 out]
            n277 = Bundle By Name(cluster=w639, "Message"="Capture Complete. Adjust the Power Supply to 3.10 volts. When ready click the capture button...", "NextState"=Gen2_FT_states."Timeout", "DUT Parameters.Batt 280"=w631) -> (w637:T6)
          }
          frame "Collect 3.1 Volts" {
            w656 = 50
            # "Average the 50 \nBattery readings"
            # "Collect the Battery readings that correspond to 3.10 volts.\nCollect the readings for 5 seconds."
            n278 = for {
              N: w656 -> [_]
              shift-right: [w662] -> w660
              shift-left: u64 0 -> [w664]
              # "Add all the Battery readings, \nso that an average can be \ncalculated later."
              # "Pull out the Battery reading from\neach set of data."
              n279 = call "RxBuffer.vi"() -> ("RxData Out"=w666:u16[])  [unwired: 8 in, 11 out]
              n280 = Wait (ms)(milliseconds to wait=u32 100) -> ()  [unwired: 1 out]
              n281 = Index Array(array=w666, index=10) -> (element=w663:u16)
              n282 = Add(x=w663, y=w664) -> (x+y=w662:u64)
            }
            n283 = Divide(x=w660, y=w656) -> (x/y=w652:dbl)
            "Batt310" <- w652
            n284 = Bundle By Name(cluster=w659, "Message"="Capture Complete. Checking Results", "NextState"=Gen2_FT_states."Battery Test", "Batt Test Step"=Batt_Cap_Steps."Check Results" ("Batt Capture State"), "DUT Parameters.Batt310"=w652) -> (w657:T6)
          }
          frame "Check Results" {
            n285 = local read "Batt280"() -> (w679:i32)
            n286 = local read "Batt310"() -> (w678:i32)
            n287 = Unbundle By Name(w681) -> ("Support Script.[[List of Errors]]"=w680:string[][], "[A/Ds]"=w668:dbl[][])
            n288 = property on="CaptureButton" class="Bool (strict)"(error in=w670, "Visible"=FALSE, "DisabledEnum"=T19."Disabled" ("Disabled")) -> (error out=w669:errorcluster)  [unwired: 1 in, 1 out]
            n289 = call "Save Batt Voltage.vi"("Battery Capture 310"=w678, "Battery Capture 280"=w679, "[A/Ds]"=w668) -> ("Pass/Fail #"=w676:i32, "Pass?"=w677:bool)  [unwired: 7 in]
            n290 = case shown="True" w677 {
              tunnel: w680 -> [w694 _]
              tunnel: w676 -> [w691 _]
              tunnel: [FALSE ("Final Program?") TRUE ("Final Program?")] -> w686
              tunnel: [Gen2_FT_states."End Test" ("NextState") Gen2_FT_states."Program Device" ("NextState")] -> w685
              tunnel: [w689 "Batt Capture successful. Attempting to reprogram the device..." ("Error Message")] -> w675
              tunnel: [w690 ""] -> w673
              tunnel: [w689 "Testing Passed" ("Error Message")] -> w672
              tunnel: [ProgramStageControl."Initial Program" ("Program Stage") ProgramStageControl."Scales" ("Program Stage")] -> w671
              frame False {
                # "Failed!"
                n291 = call "ErrorCodeDecoder.vi"("array"=w694, "FTS Error Code In"=w691) -> ("Error Message"=w689:string)
                n292 = Number To Decimal String(number=w691) -> (decimal integer string=w690:string)  [unwired: 1 in]
              }
              frame True {
                # "Passed!"
              }
            }
            n293 = local write "BatteryCapState"(0) -> ()
            n294 = Bundle By Name(cluster=w681, "Programming Mode"=w671, "NextState"=w685, "Test Result"=w686, "Message"=w675, "Final Program?"=TRUE ("Blank Device?"), "Pass/Fail #"=w673, "Result String"=w672) -> (w684:T6)
          }
        }
      }
      frame "End Test" {
        w704 = FALSE
        n295 = property on="CaptureButton" class="Bool (strict)"("Visible"=w704, "DisabledEnum"=T19."Disabled" ("Disabled"), "Value"=w704) -> ()  [unwired: 2 in, 2 out]
        n296 = property on="Shutdown Dev" class="Bool"(error in=w707, "DisabledEnum"=T19."Enabled" ("Disabled")) -> (error out=w706:errorcluster)  [unwired: 1 in, 1 out]
        n297 = property on="Start Channel:" class="CmbBox"(error in=w706, "DisabledEnum"=T19."Enabled" ("Disabled")) -> (error out=w705:errorcluster)  [unwired: 1 in, 1 out]
        n298 = call "Store Results.vi"("error in (no error)"=w705, "Data In"=w710) -> ("error out"=w711:errorcluster, "Data Out"=w709:T6)  [unwired: 8 in]
        n299 = control-ref of="Test Result"() -> (w716:refnum<vi>)
        n300 = call "Failed Test Logic.vi"("error in (no error)"=w711, "Test Result"=w716, "State-machine Local Variables in"=w709) -> ("error out"=w708:errorcluster, "Data Out"=w712:T6)  [unwired: 7 in]
        n301 = local write "Start"(FALSE ("ProgDev")) -> ()
        n302 = Bundle By Name(cluster=w712, "NextState"=Gen2_FT_states."Shutdown Device") -> (w702:T6)
      }
      frame "Display Result" {
        n303 = call "RxBuffer.vi"("error in (no error)"=w744) -> ("RxData Out"=w726:u16[], "DUT Serial Number"=→"DUT Serial Number":u32, "New Data"=w725:bool, "error out"=w743:errorcluster)  [unwired: 7 in, 8 out]
        n304 = call "BatchTest HeartBeat.vi"("MaxTime"=u32 3000, "Value In"=w725) -> ("Alive?"=w724:bool)  [unwired: 8 in, 1 out]
        n305 = call "BatchTest BoolValue Change.vi"("Value In"=w724) -> ("Value Changed?"=w742:bool, "Value Out"=w741:bool)  [unwired: 7 in, 2 out]
        n306 = First Call?() -> (First Call?: T/F=w738:bool)
        n307 = local write "Device ON?"(w724) -> ()
        n308 = Unbundle By Name(w723) -> ("DUT Parameters.Batt310"=w721:u16, "DUT Parameters.Batt 280"=w720:u16)
        n309 = Or(x=w742, y=w738) -> (x .or. y?=w739:bool)
        n310 = Index Array(array=w726, index=10) -> (element=w722:u16)
        "ADBatt" <- w722
        n311 = Array Subset(array=w726, index=3) -> (→"RawData":u16[])  [unwired: 1 in]
        n312 = case shown="True" w739 {
          tunnel: w741 -> [_ w755]
          frame False {
          }
          frame True {
            n313 = local read "Start"() -> (w754:bool)
            n314 = And(x=w755, y=w754) -> (x .and. y?=w753:bool)
            n315 = case shown="False" w753 {
              tunnel: w755 -> [w756 w757]
              frame False {
                # "Can Trigger Value Signaling"
                # "If Device is OFF or Test is OFF"
                n316 = property on="Device ON?" class="Bool (strict)"("Val(Sgnl)"=w756) -> ()  [unwired: 2 in, 2 out]
              }
              frame True {
                # "Can turn on LED only"
                # "Test is ON AND Device is ON"
                n317 = local write "Device ON?"(w757) -> ()
              }
            }
          }
        }
        n318 = local write "Batt280"(w720) -> ()
        n319 = local write "Batt310"(w721) -> ()
        n320 = call "Mark10.vi"("Data In"=w723, "error in (no error)"=w743, "Action"=Mark10_states."Read Status") -> ("Live Load"=w736:dbl, "Live Position"=w733:dbl, "error out"=w730:errorcluster)  [unwired: 12 in, 2 out]
        n321 = case shown="Error" w730 {
          selector: w730 -> [w746 _]
          tunnel: w736 -> [w748 w752]
          tunnel: [w748 w752] -> w735
          tunnel: [w747 w751] -> w734
          tunnel: w733 -> [w747 w751]
          tunnel: [w746 errorcluster {"status"=FALSE, "code"=0, "source"=""} ("error IO")] -> w732
          tunnel: [_ "Issue with Mark-10.\nMake sure unit is on and \ntry again. " ("Message")] -> w731
          frame No Error {
          }
          frame Error {
            # "Don't need Mark-10 for Battery Calc version 6/27/14 TEL\nRemoved wire to message."
          }
        }
        n322 = call "Calc Battery.vi"("Batt 280"=w720, "Batt310"=w721, "AD"=w722) -> ("Batt Volt"=→"BattVolts":dbl)  [unwired: 8 in]
        n323 = Bundle By Name(cluster=w723, "G.Load"=w735, "G.Position"=w734, "Message"=w731) -> ()  [unwired: 1 out]
      }
      frame "Exit" {
        w766 = FALSE  # Blast?
        n324 = local read "Device ON?"() -> (w762:bool)
        n325 = call "Shutdown DUT.vi"("error in (no error)"=w765, "Device On?"=w762, "Blast?"=w766, "Data In"=w764) -> ("error out"=w760:errorcluster, "State-machine Local Variables out"=w763:T6)  [unwired: 6 in]
        n326 = flat-sequence {
          tunnel: w760 -> [w767]
          tunnel: [w767] -> w759
          frame #0 {
            n327 = local write "Close Xsceiver"(TRUE ("Close Xsceiver")) -> ()
          }
        }
      }
    }
    n328 = call <vilib>:"Clear Errors.vi"("error in (no error)"=w28) -> ("error out"=w22:errorcluster)  [unwired: 6 in]
  }
  n329 = Wait on Occurrence(2:w15, 3:25000 ("ms timeout (-1)")) -> (0:w4:bool)  [unwired: 1 in]
  n330 = while {
    shift-right: [w769] -> w16
    shift-left: w3 -> [w773]
    tunnel: w4 -> [_]
    stop <- "Close Xsceiver" stop-if-true
    n331 = global read "Gen2 FT Globals.vi" "RawRxTx"() -> (w772:bool)
    n332 = case shown="False" w772 {
      tunnel: w773 -> [w775 w784]
      tunnel: [w774 w784] -> w770
      frame False {
        n333 = case shown="True" "ClearBuffer" {
          tunnel: w775 -> [w779 w782]
          tunnel: [w779 w781] -> w777
          frame False {
          }
          frame True {
            n334 = local write "ClearBuffer"(FALSE ("ClearBuffer")) -> ()
            n335 = call "RxTx.vi"("error in (no error)"=w782, "Action"=XceiverStates."Clear Buffer") -> ("error out"=w781:errorcluster)  [unwired: 9 in, 8 out]
          }
        }
        n336 = call "RxTx.vi"("error in (no error)"=w777, "Action"=XceiverStates."Rx") -> ("error out"=w774:errorcluster)  [unwired: 9 in, 8 out]
      }
      frame True {
        n337 = Wait (ms)(milliseconds to wait=u32 100) -> ()  [unwired: 1 out]
      }
    }
    n338 = call <vilib>:"Clear Errors.vi"("error in (no error)"=w770) -> ("error out"=w769:errorcluster)  [unwired: 6 in]
  }
  n339 = call "RxTx.vi"("error in (no error)"=w16, "Action"=XceiverStates."Close") -> ("error out"=w2:errorcluster)  [unwired: 9 in, 8 out]
  n340 = Merge Errors(w2, w17) -> (w13:errorcluster)
  n341 = call <vilib>:"Clear Errors.vi"("error in (no error)"=w13) -> ("error out"=w11:errorcluster)  [unwired: 6 in]
  n342 = call <vilib>:"Simple Error Handler.vi"("type of dialog (OK msg:1)"=w12, "error in (no error)"=w11) -> ("error out"=w10:errorcluster)  [unwired: 3 in, 4 out]
  n343 = disable-structure shown="RUN_TIME_ENGINE==True" {
    disable-tunnel: w10 -> [w786 w787]
    disable-tunnel: [w786 w787] -> w9
    frame condition #0 {
      n344 = Quit LabVIEW() -> ()  [unwired: 1 in]
    }
    frame condition #1 (active) {
    }
  }
  "error out" <- w9
